vi "PC_Main.vi"() -> ()   [LabVIEW 2018]
uses:
  <vilib>/Analysis/Matrix/Datatypes/RealMatrix.ctl
  controls/Command.ctl
  <vilib>/Platform/TimedLoop/XDataNode/timing_clust.ctl
  <vilib>/Platform/TimedLoop/XDataNode/nitl_modes.ctl
  <vilib>/Platform/TimedLoop/XDataNode/wakeup.ctl
  <vilib>/Utility/error.llb/DialogType.ctl
  controls/Trial Config Settings.ctl
  controls/Command IN_Recipe.ctl
  controls/Rig Config Settings.ctl
  Globals/Global - Configuration Options.vi
  <vilib>/FPGAPlugInAG/cRIO-9045/niLvFpga_Open_cRIO-9045.vi
  <vilib>/rvi/interface/common/dynamic/niFpgaDynamicAddResources.vi
  <vilib>/Utility/error.llb/Error Cluster From Error Code.vi
  <vilib>/rvi/errors/niLvFpgaAdjustHostInterfaceError.vi
  <vilib>/measure/mascope.llb/Pulse Measurements 1 chan.vi
  <vilib>/FPGAPlugInAG/Dynamic/niLvFpga_Close_Dynamic.vi
  <vilib>/Platform/TimedLoop/XDataNode/XDataNode.xnode
  <vilib>/rvi/interface/nirviOpenFPGA/nirviOpenFPGA.xnode
  FPGA Bitfiles/UIUCWhiskerProje_FPGATarget_FPGABuild_ja8qmgOJlMY.lvbitx
  FPGA_Main.vi
  <vilib>/rvi/interface/nirviMethod/nirviMethod.xnode
  <vilib>/rvi/interface/nirviCloseFPGA/nirviCloseFPGA.xnode
  <vilib>/measure/NI_MAPro.lvlib
  <vilib>/Platform/TimedLoop/XDataNode/XDNodeRunTimeDep.lvlib
  <vilib>/FPGAPlugInAG/Dynamic/niLvFpga_ReadFifo_Dynamic.vi
  <vilib>/rvi/errors/niLvFpgaMergeErrorWithErrorCode.vi
  <vilib>/Analysis/Matrix/NI_Matrix.lvlib
panel:
  out "Start Test":bool=TRUE
  out "Plot Colors OUT":u32[](array[numeric])
  in  "Tab Control 2":enum32{"Misc", "Additional Graphs"}(tab)
  in  "Flash Drive Message":string="Reading Flash Drive...."
  in  "Water Delivery":bool
  in  "Water ON Time":i32=100
  out "# water":i32
  out "Watchdog Status":string
  out "# of CPUs":u32
  out "cRIO System Time":string
  out "cRIO System Date":string
  out "Real-Time Running?":bool caption="*Flashing LED means\nreal-time status is good"
  in  "Tree":string(tree)
  in  "Open Flash Drive Directory":bool
  in  "Refresh Tree":bool
  out "Test Folder":string
  in  "Slide":dbl(slide) min=-0.1 max=1.0 step=0.0025 scale=-0.1..1.0 scale format="%.3f"
  out "Histogram":dynamicdata(graph)
  out "XY Graph":cluster{dbl[], "Array 2":dbl[]}[](graph)
  in  "Histogram Plot2":u16(ring) items=["Habituation_20.dat"]
  in  "Histogram Plot1":u16(ring) items=["Habituation_20.dat"]
  out "Active Plots":i32
  in  "Enable Histogram?":bool=TRUE
  out "Lateral Trial History":dbl[][](array[numeric])
  in  "Save Data":bool=TRUE
  out "Drive Reconnect Message":string
  in  "Log Event":bool
  in  "View Event Log":bool
  in  "Error IN":errorcluster
  out "Error Out":errorcluster
  out "User Event":refnum<user-event>
  in  "Command":T1
  out "Status":string="Please Wait....."
  in  "Tab Control":T2(tab)
  in  "Group Size for Randomization":i32=1 min=1
  in  "Randomize Trials?":bool=TRUE
  in  "Load Default Sequence":bool
  in  "Save Trial Sequence":bool
  in  "Test Trials to Run":string[](array[combo])=["Left Turn.dat", "Right Turn.dat", "Straight.dat"]
  in  "Reset Sequence to Default":bool
  in  "History (Seconds):":dbl=20.0 format="%.1f"
  in  "X Axis (Seconds):":dbl=6.0 format="%.1f"
  out "Timeout Timer":dbl format="%.2f"
  out "cor_pos":sgl format="%.3f"
  out "cor_width":sgl
  out "Trial #":i32
  in  "Save Rig Sequence":bool
  in  "Test Rig Settings":string[](array[combo])=["Left Turn.dat", "Right Turn.dat", "Straight.dat"]
  in  "Rig editor":bool
  in  "Run #":string="02"
  in  "Animal #":string="0324810"
  in  "Date":string
  in  "Start Test":bool
  in  "Trial editor":bool
  out "Time Into Trial":dbl=4.01791524887085 format="%.2f"
  in  "Graph Update Interval":dbl=0.1 format="%.2f"
  out "Chart Ball Speed":cluster{dbl[], dbl[]}[](graph) caption="Ball Speed (Vball)"
  out "Test Trial In Progress":string
  out "Trial Tracker":string[][](table)=[["Test Reward.dat", "9", "8"], ["Test NO Reward.dat", "8", "0"]]
  out "Test In Progress":bool
  out "Trial Fraction":dbl format="%.6f"
  out "Total Test Time":dbl=4.01791524887085 format="%.2f"
  out "Graph X and Y Pos":cluster{"X":dbl, "Y":dbl}[](graph) caption="X and Y Position"
  out "Speed_Time_Length":i32
  out "mean_lat_vel":dbl
  out "mean_for_vel":dbl
  out "Vball":dbl format="%.3f"
  out "A_calib_matrix":T3
  out "for_ball_motion":dbl
  out "lat_ball_motion":dbl
  out "zero_V":T3
  out "cam_vel_ai_vlt":T3
  out "cam_vel_steps":T3
  out "step_V":dbl
  out "Frame Clock":waveform(i16)(graph)
  out "Freq":dbl caption="Hz"
  in  "Frame Clock Freq":dbl=500.0 caption="Hz"
  in  "laser_ON Time":i16=1 min=0
  in  "laser_OFF Time":i16=99 min=0
  in  "Digital Controls":bool[](array[boolean])=[FALSE, FALSE, FALSE, FALSE, FALSE, FALSE]
  in  "Send Digital Signals to FPGA":bool
  in  "Ephys Clock Freq":dbl=10000.0 caption="Hz"
  in  "Manual Override":bool
  in  "Analog Inputs_Override":sgl[](array[slide]) scale=-10.0..30.0
  out "LeftWall":dbl(slide)
  out "RightWall":dbl(slide) scale=0.0..25.0
  out "Cor_width_actual":dbl
  out "cor_width 2":sgl
  out "DIO":bool[](array[boolean])
  in  "Analog Outputs":sgl[](array[numeric])=[0.0, 0.0, 0.0, 0.0] min=0 max=5 format="%.5f"
  out "Analog Inputs":sgl[](array[numeric]) format="%.5f"
  in  "Exit":bool
  # "Behavioral Control Program v1.0.0.7"
  # "Default is 10Hz"
  # "Water Delivery"
  # "Real-Time OS"
  # "ms"
  # "File Name Variables"
  # "Trial Status"
  # "Mouse Speed"
  # "Trial Config"
  # "Mouse Lateral Position"
  # "Rig Config"
  # "Mouse Forward Position"
  # "*Change this setting via Rig Editor"
  # "secs"
  # "mm"
  # "mm"
  # "secs"
  # "secs"
  # "secs"
  # "*If Speed_Time_Length = 250\nthen averages are calculated every\n0.5 seconds since 1 data save takes\nplace every 0.002 seconds."
  # "="
  # "="
  # "avg"
  # "mean_for_vel"
  # "for_ball_motion (speed_time_length)"
  # "="
  # "="
  # "avg"
  # "mean_lat_vel"
  # "lat_ball_motion (speed_time_length)"
  # "cm/s"
  # "cm/s"
  # "2"
  # "2"
  # "="
  # "+"
  # "for_ball_motion"
  # "lat_ball_motion"
  # "cm/s"
  # "A_calib(0,0) x cam_vel_steps(0)"
  # "="
  # "A_calib(0,1) x cam_vel_steps(1)"
  # "cm/s"
  # "sum"
  # "A_calib(0,2) x cam_vel_steps(2)"
  # "A_calib(0,3) x cam_vel_steps(3)"
  # "A_calib(1,0) x cam_vel_steps(0)"
  # "="
  # "A_calib(1,1) x cam_vel_steps(1)"
  # "cm/s"
  # "sum"
  # "A_calib(1,2) x cam_vel_steps(2)"
  # "A_calib(1,3) x cam_vel_steps(3)"
  # "minus"
  # "="
  # "round"
  # "trial_ephys_ctrl"
  # "*this will trigger ephys_clock"
  # "whisker_video_ctrl"
  # "*this will trigger frame_clock"
  # "right_texture_ctrl"
  # "left_texture_ctrl"
  # "water_valve_ctrl"
  # "ON Time(msec)"
  # "OFF Time(msec)"
  # "laser_ctrl"
  # "*this will cycle the laser"
  # "laser"
  # "*this will cycle the laser voltage to the\namplitude called for using the analog\noutput labeled \"laser_AO3\" which is\nlocated on the Debug tab."
  # "Forward"
  # "Lateral"
  # "ANALOG OUTPUTS - Slot2"
  # "DIGITAL IO - Slot3"
  # "ANALOG INPUTS - Slot1"
  # "Chassis:  cRIO-9045"
  # "DIO0"
  # "aClck_DI"
  # "DIO1"
  # "frame_clock_DO"
  # "whisker_video_ctrl_DO"
  # "DIO2"
  # "DIO3"
  # "lick_signal_DO"
  # "water_valve_ctrl_DO"
  # "DIO4"
  # "DIO5"
  # "laser_ctrl"
  # "DIO6"
  # "left_texture_ctrl_DO"
  # "right_texture_ctrl_DO"
  # "DIO7"
  # "DIO8"
  # "trial_ephys_ctrl_DO"
  # "trial_iti_ctrl_DO"
  # "DIO9"
  # "trial_on_ctrl_DO"
  # "DIO10"
  # "ephys_clock_DO"
  # "DIO11"
  # "NI9403"
  # "left_wall_AO0"
  # "Vdc"
  # "right_wall_AO1"
  # "Vdc"
  # "AO2"
  # "Vdc"
  # "laser_AO3"
  # "Vdc"
  # "Vx0 raw Cam0"
  # "Vdc"
  # "Vdc"
  # "Vy0 raw Cam0"
  # "Vdc"
  # "Vx1 raw Cam1"
  # "Vy1 raw Cam1"
  # "Vdc"
  # "Software Installations"
  # "Flash Drive Setup"
  # "1) Labview 2018 w/f1 patch (32-bit)\n2) 2018 Labview Real-Time Module (32-bit)\n3) 2018 Labview FPGA Module (32-bit)\n4) DAQmx 18.0\n5) NI Compact RIO Drivers 18.1 (June 2018)\n6) 2018 XILINX 2017_2 (Compile Tools)"
  # "1) Make sure a fat32 formatted flash drive is inserted into the cRIO.\n\n2) Make sure the cRIO is mapped as a network drive on the main PC (see fig.1 below).  Webdav needs to be installed on the cRIO in order to do this. \n\n3) Make sure the correct path is entered in the Rig Config Settings for \"cRIO Test Data Dir\".  The flash drive will always be \"u\".  So, if the cRIO is mapped as network drive U then the correct path to put in the Rig Config Settings would be \"U:\\u\".\n\n4) Make sure the mapped network drive path is connected (figure 1).  If it isn't you will have to double click on the path at which point a login window will pop up.  Enter your Admin login and password.  If you do not have one then create one on the cRIO using via the \"Web Configuration\" page.  The default login for the cRIO is:   User name:  \"admin\"\n                                                                                                                 Password:  blank"
  # "*Install the above software packages in the order listed."
  # "Required Directories"
  # "C:\\Whisker Tester\\Rig\\\n*This directory will include 1) rig setup files (.dat) and 2) a default rig file (Sequence.xls) \n\nC:\\Whisker Tester\\Trials\\\n*This directory will include 1) trial setup files (.dat) and 2) a default trials list (Sequence.xls) \n\nC:\\Whisker Tester\\Event Logs\\\n*This directory will include event logs for various events that the developer wants to track (log.xls)"
  # "Figure 1 - cRIO Mapped Network Drive"
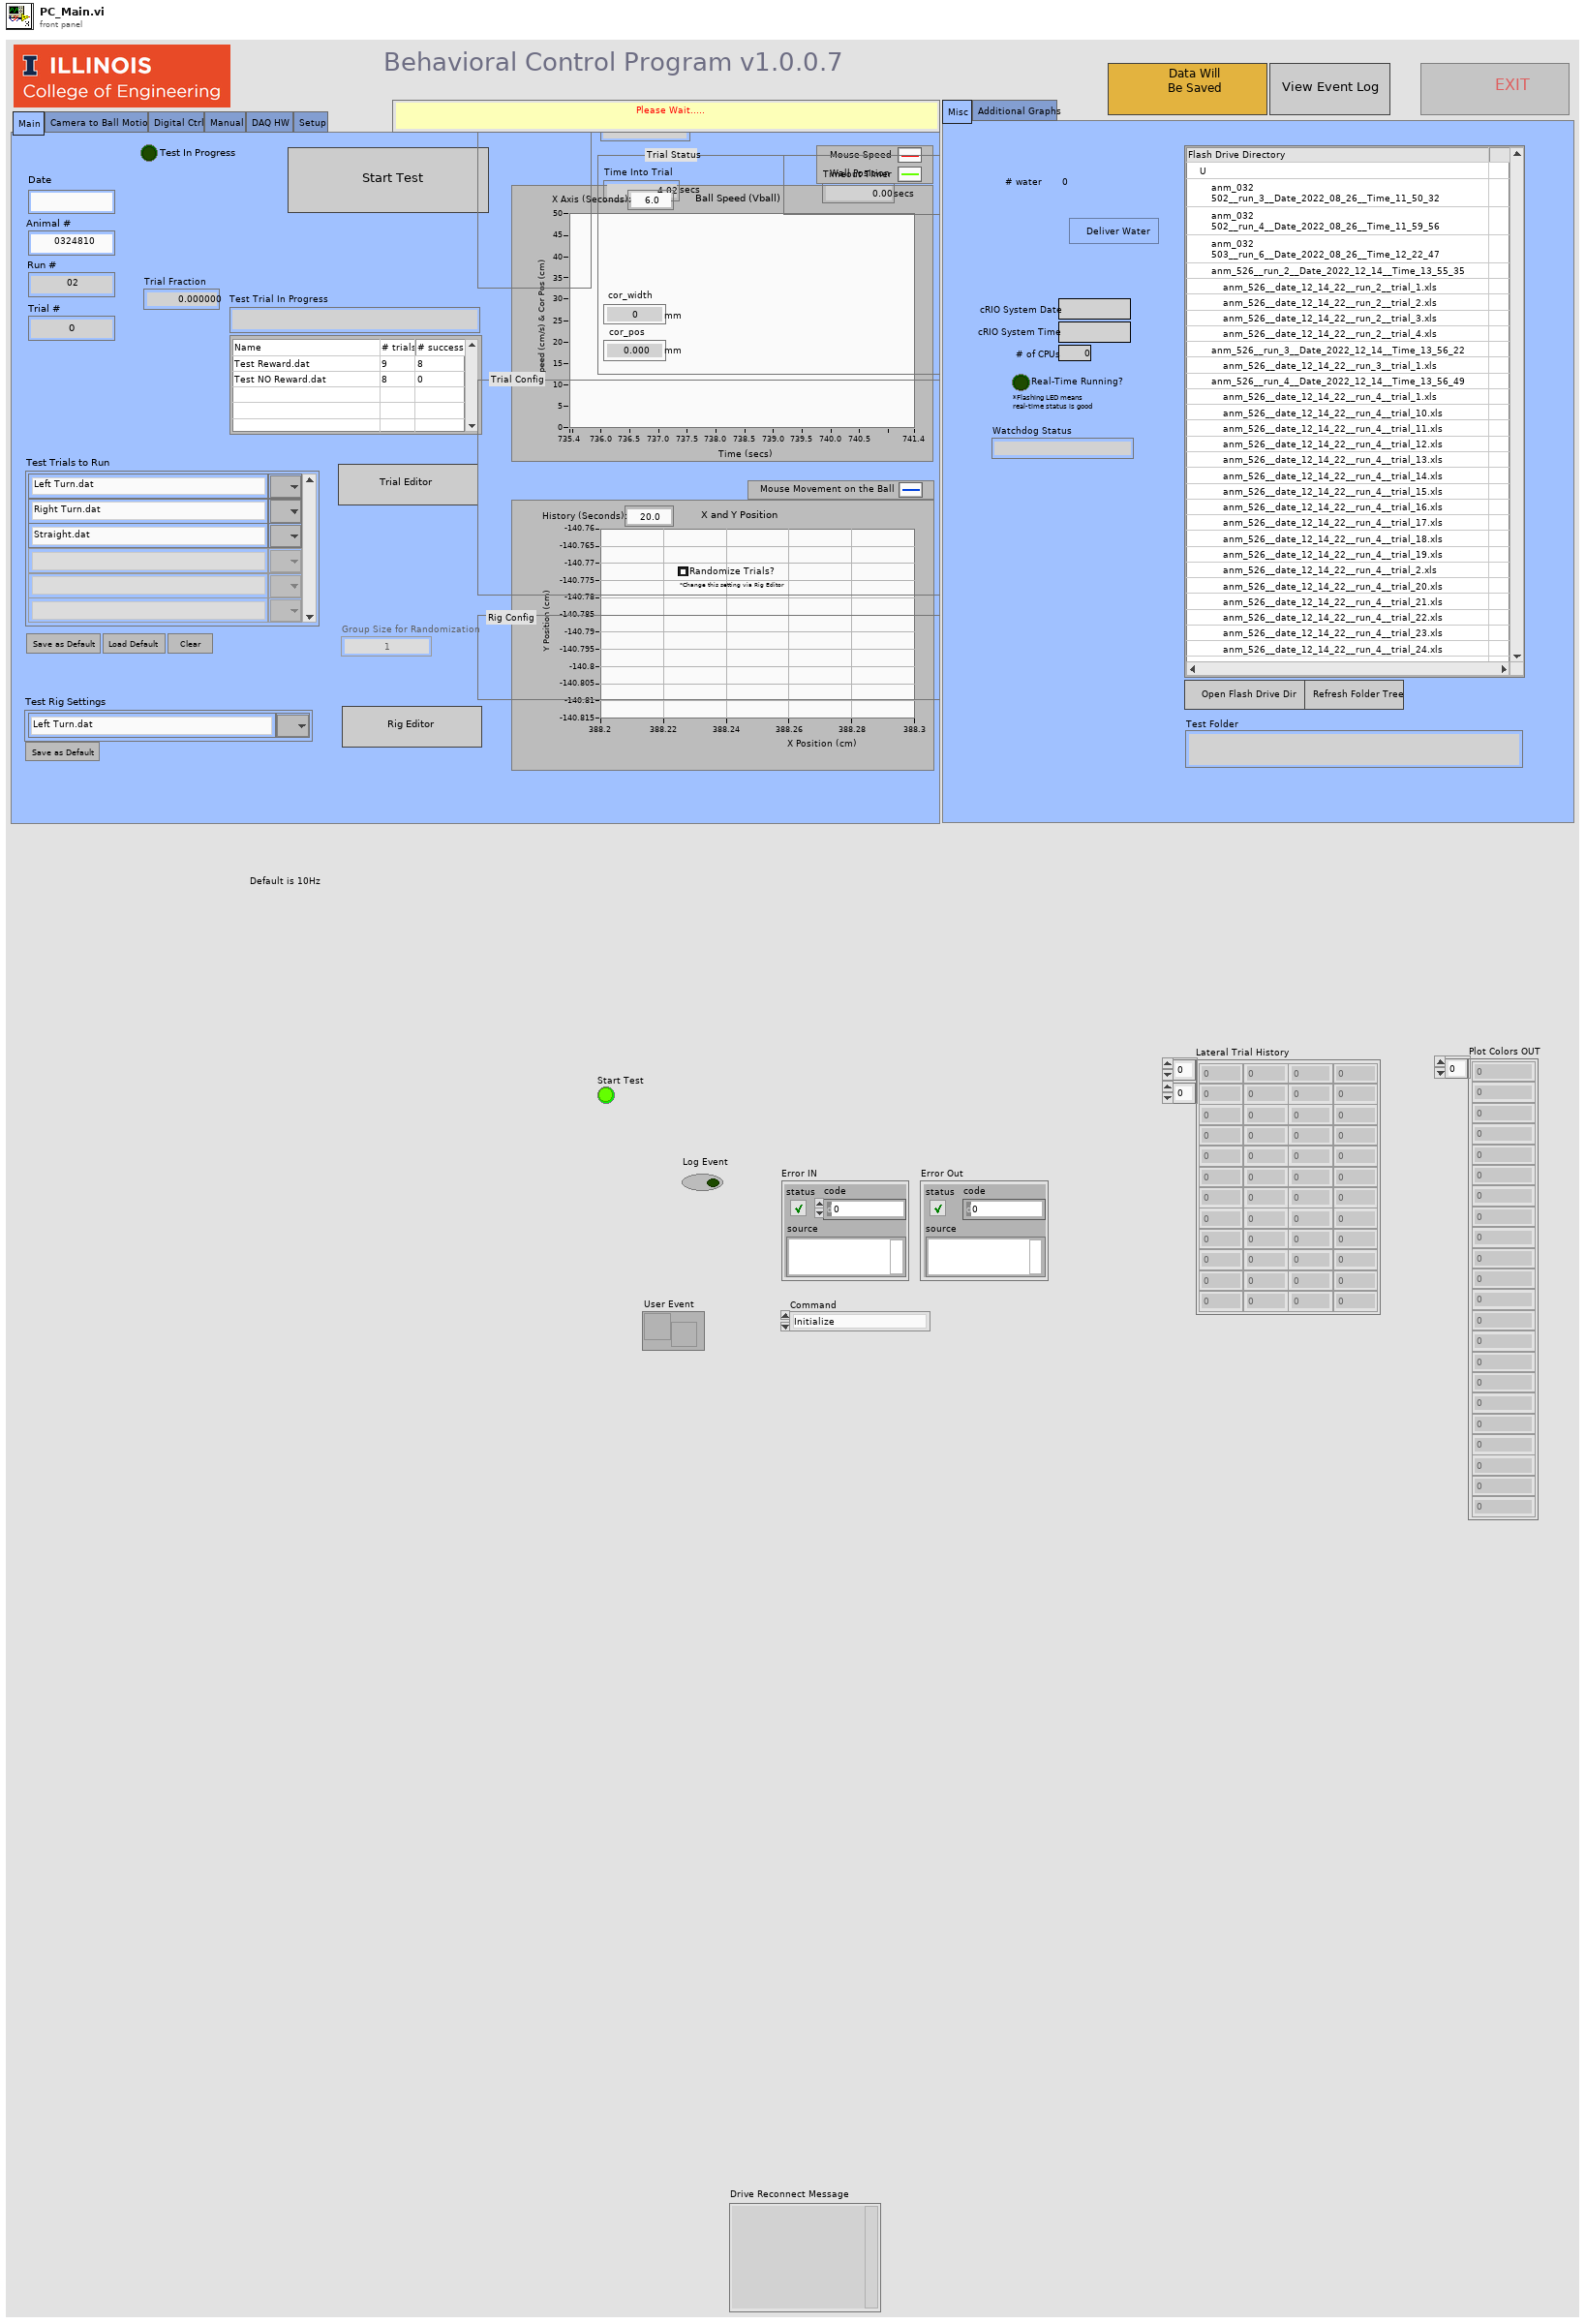
[diagram p1: front panel]
types:
  T1 = typedef "Command.ctl" = enum16{"Initialize", "Start Test", "Download All Trials to RT", "Water Delivery", "Rig Config Read", "cRIO Test Data Directory", "Update Folder Tree", "Log Event", "Abort", "Exit"}
  T2 = enum32{"Main", "Camera to Ball Motion", "Digital Ctrl", "Manual", "DAQ HW", "Setup"}
  T3 = typedef "NI_Matrix.lvlib/RealMatrix.ctl" = dbl[][]
  T4 = enum8{"Enabled", "Disabled", "Disabled and Grayed Out"}
  T5 = typedef "XDNodeRunTimeDep.lvlib/timing_clust.ctl" = cluster{"Expected End [f-1]":u64, "Actual End [f-1]":u64, "Finished Late? [f-1]":bool, "Expected End [i-1]":u64, "Actual End [i-1]":u64, "Finished Late? [i-1]":bool, "Expected Start [i]":u64, "Actual Start [i]":u64, "Expected Start [f]":u64, "Actual Start [f]":u64, "Source Name":string, "Structure Name":string, "Period":i64, "Deadline":i64, "Offset":i64, "Start":i64, "Priority":i32, "Timeout":i32, "Mode":T6, "Wakeup Reason":T7, "Error":errorcluster, "Source Type":string, "Secondary Source Type":string, "Global End Time":u64, "Global Start Time":u64, "Frame Duration":u64, "Iteration Duration":u64, "Assigned CPU":i32, "I/O Scan Engine Mode":u32}
  T6 = typedef "XDNodeRunTimeDep.lvlib/nitl_modes.ctl" = enum32{"No Change", "Process missed periods, maintain original phase", "Discard missed periods, maintain original phase", "Process missed periods, ignore original phase", "Discard missed periods, ignore original phase"}
  T7 = typedef "XDNodeRunTimeDep.lvlib/wakeup.ctl" = enum32{"Normal", "Aborted", "Asynchronous wakeup", "Timing source error", "Timed loop error", "Timeout"}
  T8 = typedef "Command IN_Recipe.ctl" = enum16{"Save", "Load"}
  T9 = enum32{"Page Enabled", "Page Disabled", "Page Disabled & Grayed"}
  T10 = enum32{"invalid app kind", "Development System", "Run Time System", "Student Edition", "Embedded LabVIEW", "Evaluation", "Custom"}
  T11 = typedef "DialogType.ctl" = u16
  T12 = typedef "Rig Config Settings.ctl" = cluster{"Rig Name":string, "Rig Room":string, "Base Directory":string, "Computer IP Address":string, "Globals Name":string, "Treatmill Str":string, "cRIO Test Data Dir":path, "ai":string, "ao":string, "dio":string, "A_calib_str_row1":string, "A_calib_str_row2":string, "A_calib_str_row3":string, "Zero_V_str":string, "step_V":string, "Sample Freq":string, "ai_threshold":string, "run_speed_thresh":string, "speed_time_length":string, "wall ball gain":string, "max wall pos":string, "max cor width":string, "Trial Config Directory":path, "Randomize Trials?":bool}
  T13 = typedef "Trial Config Settings.ctl" = cluster{"Trial Label":string, "Type":string, "Timeout (secs)":string, "Inter-Trial Interval (secs)":string, "Left Wall Enabled":bool, "Right Wall Enabled":bool, "Corridor Reset":bool, "Default Wall Position":string, "Open Loop Change Positions":string, "Open Loop Values (mm)":string, "Corridor Width Change Positions":string, "Corridor Width Values (mm) ":string, "Turn Change Positions":string, "Turn Values (deg)":string, "Left Texture Change Positions":string, "Right Texture Change Positions":string, "Video Frames (fps)":string, "Water Enabled":bool, "Water Trial Position":string, "Photostimulation":string, "Water Corridor Max":string, "Water Range":string, "Water Drop Size (ms)":string, "Water Reward Position":string, "Duration (cm)":string, "Left Texture Enabled":bool, "Right Texture Enabled":bool, "Ps Trial Period":string, "Ps Inter-Pulse-Interval (ms)":string, "Ps Peak Power":string, "Ps Pulse Duration (ms)":string, "ephys_clock freq (hz)":string, "frame_clock (hz)":string, "Plot Color (Lateral Dist vs Trial Fraction)":u32}
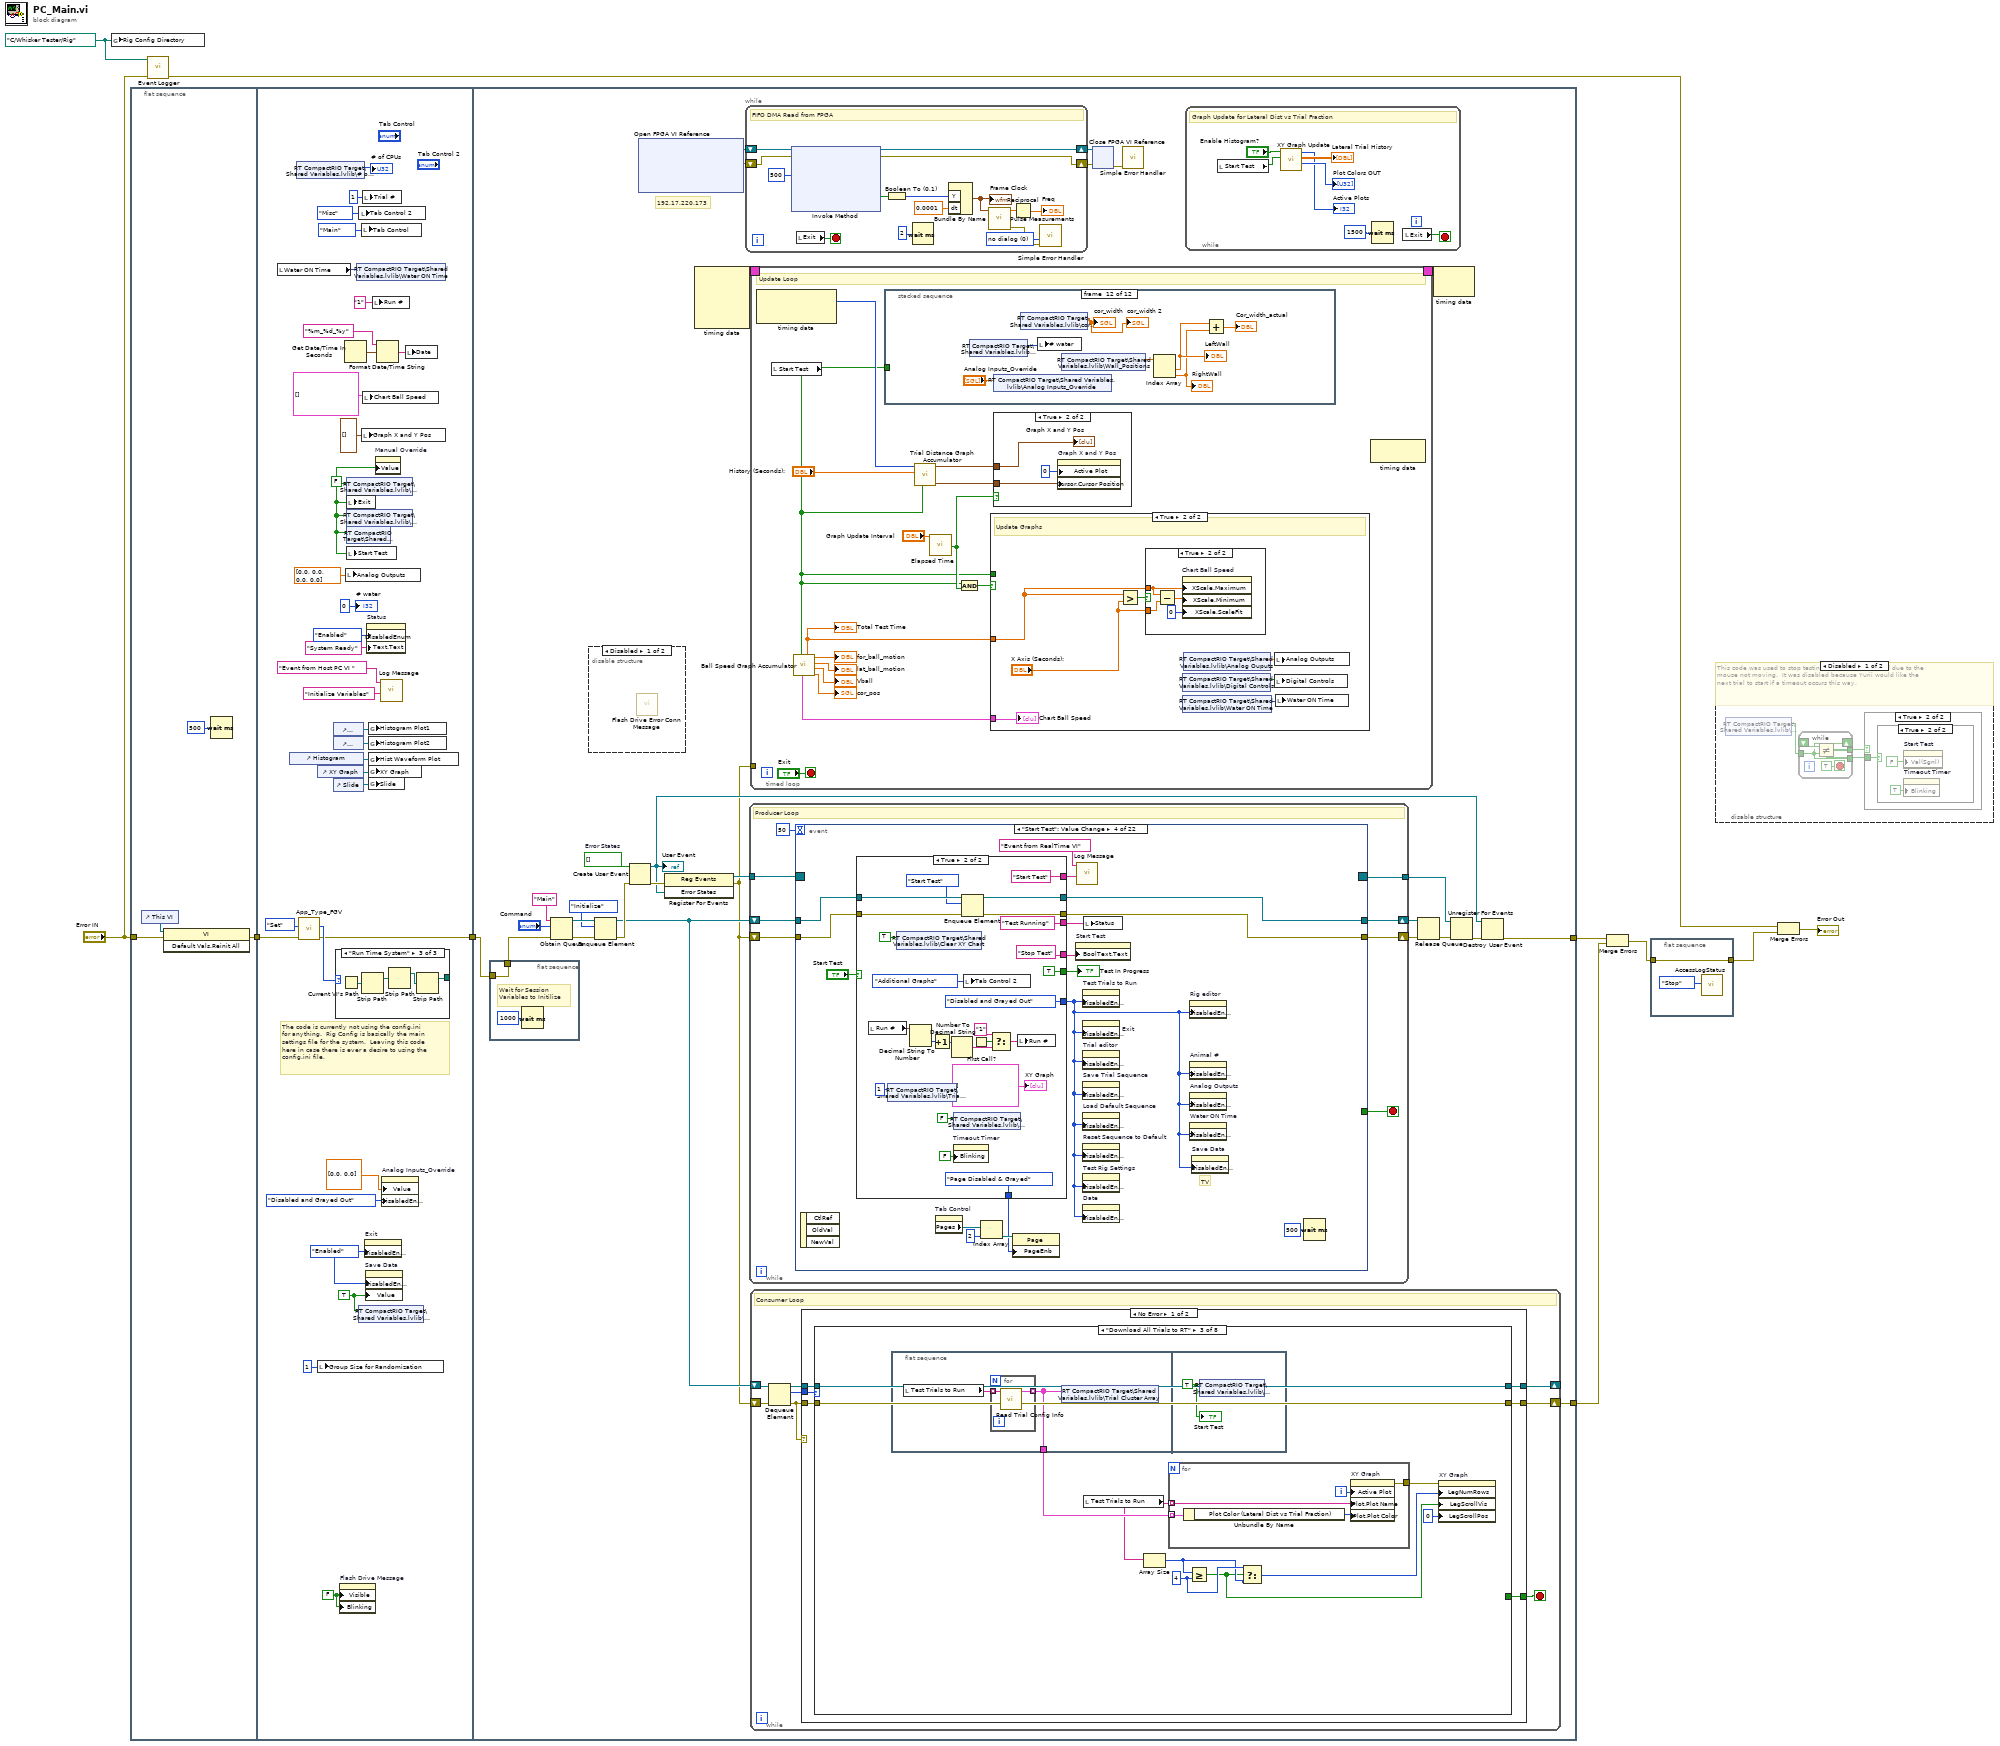
[diagram p0: block diagram]
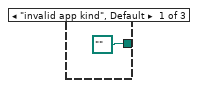
[diagram p5: hidden frame]
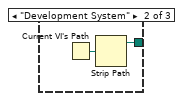
[diagram p6: hidden frame]
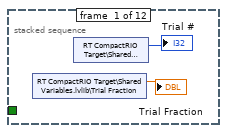
[diagram p8: hidden frame]
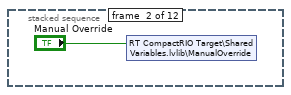
[diagram p9: hidden frame]
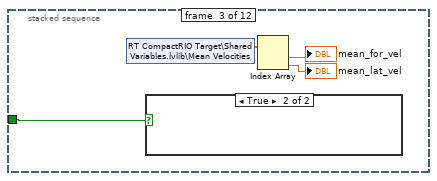
[diagram p10: hidden frame]
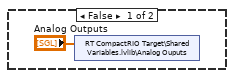
[diagram p11: hidden frame]
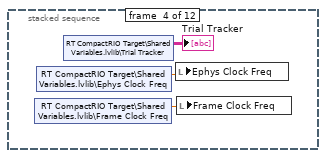
[diagram p12: hidden frame]
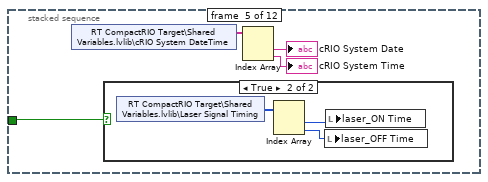
[diagram p13: hidden frame]
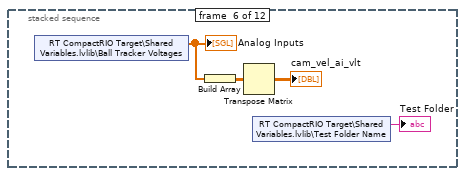
[diagram p15: hidden frame]
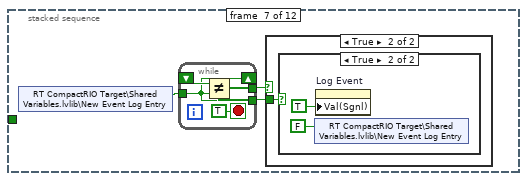
[diagram p16: hidden frame]
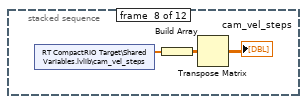
[diagram p19: hidden frame]
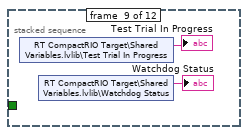
[diagram p20: hidden frame]
diagram:
  w5 = path "C:/Whisker Tester/Rig" ("Rig Config Directory")
  n1 = global write "Global - Configuration Options.vi" "Rig Config Directory"(w5) -> ()
  n2 = flat-sequence {
    tunnel: "Error IN" -> [w13]
    tunnel: [w12] -> w7
    tunnel: [w32] -> w8
    tunnel: w7 -> [w34]
    tunnel: [w66] -> w10
    tunnel: [w65] -> w9
    tunnel: w8 -> [w63]
    frame #0 {
      n3 = control-ref of="This VI"() -> (w14:refnum<vi>)
      n4 = invoke class="VI" method="Default Vals.Reinit All"(reference=w14, error in=w13) -> (error out=w12:errorcluster)  [unwired: 1 in, 2 out]
      n5 = Wait (ms)(milliseconds to wait=u32 500) -> ()  [unwired: 1 out]
    }
    frame #1 {
      w24 = FALSE ("Visible")
      w17 = T4."Enabled" ("Disabled")
      w16 = TRUE ("Save Data")
      w15 = FALSE ("New Trial Ready")
      # "The code is currently not using the config.ini\nfor anything.  Rig Config is basically the main\nsettings file for the system.  Leaving this code\nhere in case there is ever a desire to using the\nconfig.ini file."
      n6 = local read "Water ON Time"() -> (w44:i32)
      n7 = control-ref of="Histogram"() -> (w21:refnum<vi>)
      n8 = shared-variable "RT CompactRIO Target\\Shared Variables.lvlib\\# of CPUs"() -> (→"# of CPUs":u32)  [unwired: 1 in, 1 out]
      n9 = call "App_Type_FGV.vi"("error in"=w34, "Function"=enum16{"Get", "Set"}."Set") -> ("error out"=w32:errorcluster, "App. Type"=w33:T10)  [unwired: 8 in]
      n10 = control-ref of="XY Graph"() -> (w20:refnum<vi>)
      n11 = local write "Group Size for Randomization"(1 ("Group Size for Randomization")) -> ()
      n12 = control-ref of="Histogram Plot1"() -> (w22:refnum<vi>)
      n13 = control-ref of="Histogram Plot2"() -> (w23:refnum<vi>)
      n14 = control-ref of="Slide"() -> (w19:refnum<vi>)
      n15 = case shown="\"Run Time System\"" w33 {
        tunnel: [path "" ("stripped path") w49 w51] -> _
        frame "invalid app kind", Default {
        }
        frame "Development System" {
          n16 = Current VI's Path() -> (path=w50:path)
          n17 = Strip Path(path=w50) -> (stripped path=w49:path)  [unwired: 1 out]
        }
        frame "Run Time System" {
          n18 = Current VI's Path() -> (path=w52:path)
          n19 = Strip Path(path=w52) -> (stripped path=w53:path)  [unwired: 1 out]
          n20 = Strip Path(path=w53) -> (stripped path=w54:path)  [unwired: 1 out]
          n21 = Strip Path(path=w54) -> (stripped path=w51:path)  [unwired: 1 out]
        }
      }
      n22 = property on="Flash Drive Message" class="Str"("Visible"=w24, "Blinking"=w24) -> ()  [unwired: 2 in, 2 out]
      n23 = Get Date/Time In Seconds() -> (seconds since 1Jan1904=w47:timestamp)
      n24 = local write "Analog Outputs"(sgl[] [0.0, 0.0, 0.0, 0.0] ("Analog Outputs")) -> ()
      n25 = shared-variable "RT CompactRIO Target\\Shared Variables.lvlib\\Start Test"(w15) -> ()  [unwired: 1 in, 1 out]
      n26 = local write "Exit"(w15) -> ()
      n27 = shared-variable "RT CompactRIO Target\\Shared Variables.lvlib\\Timeout?"(w15) -> ()  [unwired: 1 in, 1 out]
      n28 = shared-variable "RT CompactRIO Target\\Shared Variables.lvlib\\Exit"(w15) -> ()  [unwired: 1 in, 1 out]
      n29 = local write "Start Test"(w15) -> ()
      n30 = shared-variable "RT CompactRIO Target\\Shared Variables.lvlib\\Water ON Time"(w44) -> ()  [unwired: 1 in, 1 out]
      n31 = local write "Tab Control 2"(enum32{"Misc", "Additional Graphs"}."Misc" ("Tab Control 2")) -> ()
      n32 = shared-variable "RT CompactRIO Target\\Shared Variables.lvlib\\SaveData"(w16) -> ()  [unwired: 1 in, 1 out]
      n33 = local write "Tab Control"(T2."Main" ("Tab Control")) -> ()
      n34 = local write "Graph X and Y Pos"(cluster{"X":dbl, "Y":dbl}[] [] ("XY Graph")) -> ()
      n35 = local write "Trial #"(1 ("Trial #")) -> ()
      n36 = local write "Chart Ball Speed"(cluster{dbl[], dbl[]}[] [] ("Chart Ball Speed")) -> ()
      n37 = property on="Exit" class="Bool (strict)"("DisabledEnum"=w17) -> ()  [unwired: 2 in, 2 out]
      n38 = property on="Save Data" class="Bool (strict)"("DisabledEnum"=w17, "Value"=w16) -> ()  [unwired: 2 in, 2 out]
      n39 = property on="Status" class="Str"("DisabledEnum"=T4."Enabled" ("Disabled"), "Text.Text"="System Ready" ("Status")) -> ()  [unwired: 2 in, 2 out]
      n40 = global write "Global - Configuration Options.vi" "Histogram Plot1"(w22) -> ()
      n41 = global write "Global - Configuration Options.vi" "Histogram Plot2"(w23) -> ()
      n42 = global write "Global - Configuration Options.vi" "Hist Waveform Plot"(w21) -> ()
      n43 = global write "Global - Configuration Options.vi" "XY Graph"(w20) -> ()
      n44 = global write "Global - Configuration Options.vi" "Slide"(w19) -> ()
      n45 = local write "Run #"("1" ("Run #")) -> ()
      n46 = property on="Manual Override" class="Bool (strict)"("Value"=w15) -> ()  [unwired: 2 in, 2 out]
      n47 = Format Date/Time String(time format string (%c)="%m_%d_%y", seconds (now)=w47) -> (date/time string=w45:string)  [unwired: 1 in]
      n48 = call "Log Message.vi"("Message"="Initialize Variables", "Log Type"="Event from Host PC VI ") -> ()  [unwired: 8 in, 2 out]
      n49 = property on="Analog Inputs_Override" class="Arr (strict)"("Value"=sgl[] [0.0, 0.0] ("Analog Inputs_Override"), "DisabledEnum"=T4."Disabled and Grayed Out" ("Disabled")) -> ()  [unwired: 2 in, 2 out]
      n50 = local write "Date"(w45) -> ()
      "# water" <- 0 ("# water")
    }
    frame #2 {
      w70 = bool[] []  # Error States
      # "192.17.220.173"
      n51 = flat-sequence {
        tunnel: w63 -> [w192]
        tunnel: [w192] -> w62
        frame #0 {
          # "Wait for Session\nVariables to Initilize"
          n52 = Wait (ms)(milliseconds to wait=u32 1000) -> ()  [unwired: 1 out]
        }
      }
      n53 = Obtain Queue(name (unnamed)="Main", element data type="Command", error in (no error)=w62) -> (queue out=w79:refnum<queue>, error out=w78:errorcluster)  [unwired: 2 in, 1 out]
      n54 = disable-structure shown="Disabled" {
        frame Disabled {
          n55 = call "Flash Drive Error Conn Message.vi"() -> ()  [unwired: 12 in]
        }
        frame Enabled {
        }
      }
      n56 = Enqueue Element(queue=w79, element=Command."Initialize", error in (no error)=w78) -> (queue out=w68:refnum<queue>, error out=w80:errorcluster)  [unwired: 1 in, 1 out]
      n57 = Create User Event(user event datatype=w70, error in=w80) -> (user event=w71:refnum<user-event>, error out=w81:errorcluster)
      "User Event" <- w71
      n58 = xnode "Open FPGA VI Reference"() -> ("FPGA VI Reference Out"=w59:refnum<k20>, "error out"=w55:errorcluster)  [unwired: 2 in]
      n59 = register-events(error in=w81, w71) -> (reference out=w82:refnum<event-registration>, error out=w64:errorcluster)  [unwired: 1 in]
      n60 = node-c288() -> (w61:T5)  [unwired: 4 in]
      n61 = while {
        shift-right: [w94] -> w57
        shift-left: w59 -> [w97]
        shift-right: [w93] -> w56
        shift-left: w55 -> [w92]
        stop <- w96 stop-if-true
        w84 = T11 0 items=["no dialog", "OK message", "continue or stop message", "OK message + warnings", "continue/stop + warnings"] ("type of dialog (OK msg:1)")
        # "FIFO DMA Read from FPGA"
        n62 = xnode "Invoke Method"("FPGA VI Reference In"=w97, "error in"=w92, "Number of Elements"=u32 500) -> ("FPGA VI Reference Out"=w94:refnum<k20>, "error out"=w93:errorcluster, "Data"=w89:bool[])  [unwired: 1 in, 1 out]
        n63 = local read "Exit"() -> (w96:bool)
        n64 = Boolean To (0,1)(Boolean=w89) -> (0, 1=w90:i16[])
        n65 = Wait (ms)(milliseconds to wait=u32 2) -> ()  [unwired: 1 out]
        n66 = Bundle By Name("Y"=w90, "dt"=0.0001) -> (w87:waveform(i16))  [unwired: 1 in]
        "Frame Clock" <- w87
        n67 = call-poly <vilib>:"Pulse Measurements.vi"("signal in"=w87) -> ("error out"=w85:errorcluster, "period"=w88:dbl)  [unwired: 6 in, 3 out]
        n68 = Reciprocal(x=w88) -> (1/x=→"Freq":dbl)
        n69 = call <vilib>:"Simple Error Handler.vi"("type of dialog (OK msg:1)"=w84, "error in (no error)"=w85) -> ()  [unwired: 3 in, 5 out]
      }
      n70 = while {
        tunnel: w82 -> [w429]
        shift-right: [w425] -> w74
        shift-left: w68 -> [w427]
        shift-right: [w424] -> w73
        shift-left: w64 -> [w426]
        tunnel: [w428] -> w72
        stop <- w430 stop-if-true
        # "Producer Loop"
        n71 = event shown="[3] \"Start Test\": Value Change" {
          selector: w429 -> [_ _ _ _ _ _ _ _ _ _ _ _ _ _ _ _ _ _ _ _ _ _]
          dyn-events: [_ _ _ _ _ _ _ _ _ _ _ _ _ _ _ _ _ _ _ _ _ _] -> w428
          timeout: 50 -> [_ _ _ _ _ _ _ _ _ _ _ _ _ _ _ _ _ _ _ _ _ _]
          tunnel: [_ _ _ _ _ _ _ _ _ _ _ _ _ _ _ _ _ _ _ _ _ TRUE] -> w430
          tunnel: w427 -> [w432 w434 w441 w458 w504 w509 w516 w522 w527 w537 w539 w542 w548 w553 w569 w572 w601 w614 w622 w625 w630 w635]
          tunnel: w426 -> [w431 w433 w440 w456 w503 w508 w515 w521 w526 w536 w538 w541 w547 w552 w566 w571 w600 w613 w621 w624 w629 w634]
          tunnel: [w432 w434 w441 w457 w504 w509 w516 w520 w527 w537 w539 w542 w548 w551 w568 w572 w601 w614 w620 w625 w630 w633] -> w425
          tunnel: [w431 w433 w440 w455 w503 w508 w514 w519 w526 w536 w538 w541 w547 w550 w567 w571 w600 w613 w619 w624 w629 w632] -> w424
          event Timeout {
            n72 = event-data() -> ()  [unwired: 1 in, 3 out]
          }
          event "Save Trial Sequence": Value Change {
            n73 = event-data() -> ()  [unwired: 1 in, 6 out]
            n74 = flat-sequence {
              frame #0 {
                n75 = call "Sequence Read_Write.vi"("Trial or Rig"=enum16{"Trial", "Rig"}."Trial", "Sequence IN"="Test Trials to Run", "Select"=enum16{"Save Sequence", "Read Sequence"}."Save Sequence") -> ()  [unwired: 7 in, 2 out]
              }
              frame #1 {
                n76 = Wait (ms)(milliseconds to wait=u32 500) -> ()  [unwired: 1 out]
              }
              frame #2 {
                n77 = local write "Save Trial Sequence"(FALSE ("Save Sequence")) -> ()
              }
            }
          }
          event "Save Rig Sequence": Value Change {
            n78 = event-data() -> ()  [unwired: 1 in, 6 out]
            n79 = flat-sequence {
              frame #0 {
                n80 = call "Sequence Read_Write.vi"("Trial or Rig"=enum16{"Trial", "Rig"}."Rig", "Sequence IN"="Test Rig Settings", "Select"=enum16{"Save Sequence", "Read Sequence"}."Save Sequence") -> ()  [unwired: 7 in, 2 out]
              }
              frame #1 {
                n81 = Wait (ms)(milliseconds to wait=u32 500) -> ()  [unwired: 1 out]
              }
              frame #2 {
                n82 = local write "Save Rig Sequence"(FALSE ("Save Sequence")) -> ()
              }
            }
          }
          event "Start Test": Value Change {
            # "TV"
            n83 = event-data() -> ()  [unwired: 1 in, 3 out]
            n84 = case shown="True" "Start Test" {
              tunnel: [T4."Enabled" ("Disabled") T4."Disabled and Grayed Out" ("Disabled")] -> w447
              tunnel: ["Start Test" ("Boolean Text.Text") "Stop Test" ("Boolean Text.Text")] -> w461
              tunnel: [FALSE ("Start Test") TRUE ("Start Test")] -> w460
              tunnel: ["Test Stopped" ("Status") "Test Running" ("Status")] -> w459
              tunnel: w458 -> [w467 w497]
              tunnel: [w465 w496] -> w457
              tunnel: w456 -> [w466 w494]
              tunnel: [w464 w493] -> w455
              tunnel: [T9."Page Enabled" ("Page Enabled State") T9."Page Disabled & Grayed" ("Page Enabled State")] -> w451
              tunnel: ["Stop Test" ("Message") "Start Test" ("Message")] -> w450
              frame False {
                n85 = stacked-sequence {
                  frame #0 {
                    w474 = FALSE ("Start Test")
                    n86 = shared-variable "RT CompactRIO Target\\Shared Variables.lvlib\\Start Test"(w474) -> ()  [unwired: 1 in, 1 out]
                    n87 = local write "Start Test"(w474) -> ()
                  }
                  frame #1 {
                    # "Give Real-Time VI time to\nhandle this manual test stop\nfrom this Host VI."
                    n88 = Wait (ms)(milliseconds to wait=u32 100) -> ()  [unwired: 1 out]
                  }
                  frame #2 {
                    w476 = bool[] [FALSE, FALSE, FALSE, FALSE, FALSE, FALSE] ("Digital Controls")
                    n89 = local write "Analog Outputs"(sgl[] [0.0, 0.0, 0.0, 0.0] ("Analog Outputs")) -> ()
                    n90 = local write "Digital Controls"(w476) -> ()
                    n91 = shared-variable "RT CompactRIO Target\\Shared Variables.lvlib\\Digital Controls"(w476) -> ()  [unwired: 1 in, 1 out]
                  }
                }
                n92 = Enqueue Element(queue=w467, element=Command."Update Folder Tree", error in (no error)=w466) -> (queue out=w465:refnum<queue>, error out=w464:errorcluster)  [unwired: 1 in, 1 out]
              }
              frame True {
                n93 = local read "Run #"() -> (w484:string)
                n94 = shared-variable "RT CompactRIO Target\\Shared Variables.lvlib\\Trial Index"(1 ("Trial Index")) -> ()  [unwired: 1 in, 1 out]
                n95 = shared-variable "RT CompactRIO Target\\Shared Variables.lvlib\\Clear XY Chart"(TRUE ("Clear XY Chart")) -> ()  [unwired: 1 in, 1 out]
                n96 = Decimal String To Number(string=w484) -> (number=w483:i32)  [unwired: 2 in, 1 out]
                n97 = Increment(x=w483) -> (x+1=w482:i32)
                n98 = Number To Decimal String(number=w482) -> (decimal integer string=w481:string)  [unwired: 1 in]
                n99 = property on="Timeout Timer" class="DigNum (strict)"("Blinking"=FALSE) -> ()  [unwired: 2 in, 2 out]
                n100 = shared-variable "RT CompactRIO Target\\Shared Variables.lvlib\\Timeout?"(FALSE ("Timeout?")) -> ()  [unwired: 1 in, 1 out]
                n101 = Enqueue Element(queue=w497, element=Command."Start Test", error in (no error)=w494) -> (queue out=w496:refnum<queue>, error out=w493:errorcluster)  [unwired: 1 in, 1 out]
                n102 = local write "Tab Control 2"(enum32{"Misc", "Additional Graphs"}."Additional Graphs" ("Tab Control 2")) -> ()
                n103 = First Call?() -> (First Call?: T/F=w487:bool)
                n104 = Select(t="1" ("Boolean Text.Text"), s=w487, f=w481) -> (s? t:f=w485:string)
                n105 = local write "Run #"(w485) -> ()
                "XY Graph" <- cluster{dbl[], "Array 2":dbl[]}[] [] ("XY Graph")
              }
            }
            "Test In Progress" <- w460
            n106 = property on="Tab Control" class="TabCtl (strict)"() -> ("Pages"=w453:refnum<vi>[])  [unwired: 2 in, 2 out]
            n107 = Index Array(array=w453, index=2) -> (element=w454:refnum<vi>)
            n108 = property class="Page"(reference=w454, "PageEnb"=w451) -> ()  [unwired: 1 in, 2 out]
            n109 = property on="Start Test" class="Bool (strict)"("BoolText.Text"=w461) -> ()  [unwired: 2 in, 2 out]
            n110 = call "Log Message.vi"("Message"=w450, "Log Type"="Event from RealTime VI") -> ()  [unwired: 8 in, 2 out]
            n111 = property on="Test Trials to Run" class="Arr (strict)"("DisabledEnum"=w447) -> ()  [unwired: 2 in, 2 out]
            n112 = property on="Exit" class="Bool (strict)"("DisabledEnum"=w447) -> ()  [unwired: 2 in, 2 out]
            n113 = property on="Trial editor" class="Bool (strict)"("DisabledEnum"=w447) -> ()  [unwired: 2 in, 2 out]
            n114 = property on="Save Trial Sequence" class="Bool (strict)"("DisabledEnum"=w447) -> ()  [unwired: 2 in, 2 out]
            n115 = property on="Load Default Sequence" class="Bool (strict)"("DisabledEnum"=w447) -> ()  [unwired: 2 in, 2 out]
            n116 = property on="Reset Sequence to Default" class="Bool (strict)"("DisabledEnum"=w447) -> ()  [unwired: 2 in, 2 out]
            n117 = property on="Test Rig Settings" class="Arr (strict)"("DisabledEnum"=w447) -> ()  [unwired: 2 in, 2 out]
            n118 = property on="Date" class="Str"("DisabledEnum"=w447) -> ()  [unwired: 2 in, 2 out]
            n119 = local write "Status"(w459) -> ()
            n120 = property on="Rig editor" class="Bool (strict)"("DisabledEnum"=w447) -> ()  [unwired: 2 in, 2 out]
            n121 = property on="Animal #" class="Str"("DisabledEnum"=w447) -> ()  [unwired: 2 in, 2 out]
            n122 = property on="Analog Outputs" class="Arr (strict)"("DisabledEnum"=w447) -> ()  [unwired: 2 in, 2 out]
            n123 = property on="Water ON Time" class="DigNum (strict)"("DisabledEnum"=w447) -> ()  [unwired: 2 in, 2 out]
            n124 = property on="Save Data" class="Bool (strict)"("DisabledEnum"=w447) -> ()  [unwired: 2 in, 2 out]
            n125 = Wait (ms)(milliseconds to wait=u32 500) -> ()  [unwired: 1 out]
          }
          event "Slide": Mouse Up {
            n126 = event-data() -> ()  [unwired: 1 in, 4 out]
            n127 = local read "Enable Histogram?"() -> (w502:bool)
            n128 = case shown="True" w502 {
              frame False {
              }
              frame True {
                n129 = shared-variable "RT CompactRIO Target\\Shared Variables.lvlib\\Test Trial Plot Color Array"() -> (w507:u32[])  [unwired: 1 in, 1 out]
                n130 = shared-variable "RT CompactRIO Target\\Shared Variables.lvlib\\Lateral Trial History"() -> (w506:dbl[][])  [unwired: 1 in, 1 out]
                n131 = call "Histogram Update.vi"("Lat Hist at Trial Fraction"=w506, "Test Trial Plot Color Array IN"=w507, "Trial Fraction Interval"=0.0025 ("y")) -> ()  [unwired: 12 in, 5 out]
              }
            }
          }
          event "Slide": Value Change {
            n132 = event-data() -> ()  [unwired: 1 in, 6 out]
            n133 = property on="XY Graph" class="XYGraph (strict)"("Active Cursor"=u32 0, "Cursor.Cursor X"="Slide", "Cursor.Cursor Y"=-10.0 ("Cursor.Cursor Position:Cursor Y")) -> ()  [unwired: 2 in, 2 out]
          }
          event "View Event Log": Value Change {
            n134 = event-data() -> ()  [unwired: 1 in, 6 out]
            n135 = call "Popup - Event Log Viewer.vi"("Error IN"=w515) -> ("Error OUT"=w513:errorcluster)  [unwired: 10 in]
            n136 = flat-sequence {
              tunnel: w513 -> [w517]
              tunnel: [w517] -> w514
              frame #0 {
                n137 = local write "View Event Log"(FALSE ("View Event Log")) -> ()
              }
            }
          }
          event "Open Flash Drive Directory": Value Change {
            n138 = event-data() -> ()  [unwired: 1 in, 6 out]
            n139 = Enqueue Element(queue=w522, element=Command."cRIO Test Data Directory", error in (no error)=w521) -> (queue out=w520:refnum<queue>, error out=w519:errorcluster)  [unwired: 1 in, 1 out]
          }
          event "Send Digital Signals to FPGA": Value Change {
            n140 = event-data() -> ()  [unwired: 1 in, 6 out]
            n141 = stacked-sequence {
              frame #0 {
                n142 = Build Array("laser_ON Time", "laser_OFF Time") -> (w532:i16[])
                n143 = shared-variable "RT CompactRIO Target\\Shared Variables.lvlib\\Ephys Clock Freq"("Ephys Clock Freq") -> ()  [unwired: 1 in, 1 out]
                n144 = shared-variable "RT CompactRIO Target\\Shared Variables.lvlib\\Frame Clock Freq"("Frame Clock Freq") -> ()  [unwired: 1 in, 1 out]
                n145 = shared-variable "RT CompactRIO Target\\Shared Variables.lvlib\\Laser Signal Timing"(w532) -> ()  [unwired: 1 in, 1 out]
              }
              frame #1 {
                n146 = Wait (ms)(milliseconds to wait=u32 500) -> ()  [unwired: 1 out]
              }
              frame #2 {
                n147 = local write "Send Digital Signals to FPGA"(FALSE ("Send Digital Signals to FPGA")) -> ()
              }
            }
            n148 = shared-variable "RT CompactRIO Target\\Shared Variables.lvlib\\Digital Controls"("Digital Controls") -> ()  [unwired: 1 in, 1 out]
            n149 = property on="Send Digital Signals to FPGA" class="Bool (strict)"("DisabledEnum"=T4."Disabled and Grayed Out" ("Disabled")) -> ()  [unwired: 2 in, 2 out]
          }
          event "Digital Controls", "Ephys Clock Freq", "Frame Clock Freq", "laser_OFF Time", "laser_ON Time": Value Change {
            n150 = event-data() -> ()  [unwired: 1 in, 6 out]
            n151 = property on="Send Digital Signals to FPGA" class="Bool (strict)"("DisabledEnum"=T4."Enabled" ("Disabled")) -> ()  [unwired: 2 in, 2 out]
          }
          event "Trial editor": Value Change {
            n152 = event-data() -> ()  [unwired: 1 in, 6 out]
            n153 = flat-sequence {
              frame #0 {
                n154 = call "Trial - Editor.vi"() -> ()  [unwired: 11 in, 1 out]
              }
              frame #1 {
                n155 = local write "Trial editor"(FALSE ("Trial editor")) -> ()
              }
            }
          }
          event "Manual Override": Value Change {
            n156 = event-data() -> ("NewVal"=w543:bool)  [unwired: 1 in, 5 out]
            n157 = case shown="False" w543 {
              frame False {
                n158 = property on="Analog Inputs_Override" class="Arr (strict)"("Value"=sgl[] [0.0, 0.0] ("Analog Inputs_Override"), "DisabledEnum"=T4."Disabled and Grayed Out" ("Disabled")) -> ()  [unwired: 2 in, 2 out]
              }
              frame True {
                n159 = property on="Analog Inputs_Override" class="Arr (strict)"("DisabledEnum"=T4."Enabled" ("Disabled")) -> ()  [unwired: 2 in, 2 out]
              }
            }
          }
          event "Save Data": Value Change {
            n160 = event-data() -> ("NewVal"=w549:bool)  [unwired: 1 in, 5 out]
            n161 = shared-variable "RT CompactRIO Target\\Shared Variables.lvlib\\SaveData"(w549) -> ()  [unwired: 1 in, 1 out]
          }
          event "Rig editor": Value Change {
            n162 = event-data() -> ()  [unwired: 1 in, 6 out]
            n163 = stacked-sequence {
              tunnel: w553 -> [_ _ w563 _]
              tunnel: w552 -> [_ _ w562 _]
              tunnel: [_ _ w561 _] -> w551
              tunnel: [_ _ w560 _] -> w550
              frame #0 {
                n164 = call "Rig - Editor.vi"() -> ()  [unwired: 11 in, 1 out]
              }
              frame #1 {
                n165 = global read "Global - Configuration Options.vi" "Rig Config Settings"() -> (w559:T12)
                n166 = Unbundle By Name(w559) -> ("Randomize Trials?"=w554:bool)
                n167 = local write "Randomize Trials?"(w554) -> ()
                n168 = Select(t=T4."Enabled" ("Disabled"), s=w554, f=T4."Disabled and Grayed Out" ("Disabled")) -> (s? t:f=w558:T4)
                n169 = property on="Group Size for Randomization" class="DigNum (strict)"("DisabledEnum"=w558, "Value"=1 ("Group Size for Randomization")) -> ()  [unwired: 2 in, 2 out]
              }
              frame #2 {
                n170 = Enqueue Element(queue=w563, element=Command."Rig Config Read", error in (no error)=w562) -> (queue out=w561:refnum<queue>, error out=w560:errorcluster)  [unwired: 1 in, 1 out]
              }
              frame #3 {
                n171 = local write "Rig editor"(FALSE ("Trial editor")) -> ()
              }
            }
          }
          event "Refresh Tree": Value Change {
            n172 = event-data() -> ()  [unwired: 1 in, 6 out]
            n173 = Enqueue Element(queue=w569, element=Command."Update Folder Tree", error in (no error)=w566) -> (queue out=w568:refnum<queue>, error out=w567:errorcluster)  [unwired: 1 in, 1 out]
          }
          event "Load Default Sequence": Value Change {
            n174 = event-data() -> ()  [unwired: 1 in, 6 out]
            n175 = stacked-sequence {
              seq-local: [w573 _ _ _] -> [_ _ _ w586]
              frame #0 {
                w578 = refnum<vi> refnum  # ComboBox
                n176 = control-ref of="Test Trials to Run"() -> (w579:refnum<vi>)
                n177 = invoke class="Arr (strict)" method="Reinit To Default"(reference=w579) -> (error out=w575:errorcluster)  [unwired: 2 in, 2 out]
                n178 = property on="Test Trials to Run" class="Arr (strict)"(error in=w575) -> (error out=w574:errorcluster, "Array Element"=w577:refnum<vi>)  [unwired: 1 in, 1 out]
                n179 = call "Trial Config - Load Filenames.vi"() -> ("Trial Config File Names OUT"=w573:string[])  [unwired: 10 in, 1 out]
                n180 = To More Specific Class(target class=w578, reference=w577) -> (specific class reference=w576:refnum<vi>)  [unwired: 1 in, 1 out]
                n181 = property class="CmbBox"(reference=w576, error in=w574, "Strings[]"=w573) -> ()  [unwired: 2 out]
              }
              frame #1 {
                n182 = Wait (ms)(milliseconds to wait=u32 500) -> ()  [unwired: 1 out]
              }
              frame #2 {
                n183 = local write "Load Default Sequence"(FALSE ("Load Default Sequence")) -> ()
              }
              frame #3 {
                # "make sure saved sequence\ncontains recipes that exist"
                n184 = call "Sequence Read_Write.vi"("Select"=enum16{"Save Sequence", "Read Sequence"}."Read Sequence") -> ("Sequence OUT"=w583:string[])  [unwired: 9 in, 1 out]
                n185 = for {
                  tunnel: w583 -> [w590] mode=indexing
                  tunnel: w586 -> [w589]
                  shift-right: [w587] -> w584
                  shift-left: string[] [] -> [w588]
                  n186 = for {
                    tunnel: w590 -> [w592]
                    tunnel: w589 -> [w595] mode=indexing
                    tunnel: w588 -> [w593]
                    tunnel: [w591] -> w587
                    stop <- w594 stop-if-true
                    n187 = Equal?(x=w592, y=w595) -> (x = y?=w594:bool)
                    n188 = case shown="True" w594 {
                      tunnel: w593 -> [w596 w599]
                      tunnel: w592 -> [_ w598]
                      tunnel: [w596 w597] -> w591
                      frame False {
                      }
                      frame True {
                        n189 = Build Array (concatenate)(w599, w598) -> (w597:string[])
                      }
                    }
                  }
                }
                n190 = local write "Test Trials to Run"(w584) -> ()
              }
            }
          }
          event "Reset Sequence to Default": Value Change {
            n191 = event-data() -> ()  [unwired: 1 in, 6 out]
            n192 = stacked-sequence {
              frame #0 {
                n193 = control-ref of="Test Trials to Run"() -> (w602:refnum<vi>)
                n194 = invoke class="Arr (strict)" method="Reinit To Default"(reference=w602) -> ()  [unwired: 2 in, 3 out]
              }
              frame #1 {
                w604 = refnum<vi> refnum  # ComboBox
                n195 = property on="Test Trials to Run" class="Arr (strict)"() -> ("Array Element"=w605:refnum<vi>)  [unwired: 2 in, 2 out]
                n196 = call "Trial Config - Load Filenames.vi"() -> ("Trial Config File Names OUT"=w603:string[])  [unwired: 10 in, 1 out]
                n197 = To More Specific Class(target class=w604, reference=w605) -> (specific class reference=w606:refnum<vi>)  [unwired: 1 in, 1 out]
                n198 = property class="CmbBox"(reference=w606, "Strings[]"=w603) -> ()  [unwired: 1 in, 2 out]
              }
              frame #2 {
                n199 = local write "Test Trials to Run"(string[] [] ("Test Trials to Run")) -> ()
              }
              frame #3 {
                n200 = Wait (ms)(milliseconds to wait=u32 500) -> ()  [unwired: 1 out]
              }
              frame #4 {
                n201 = local write "Reset Sequence to Default"(FALSE ("Reset Sequence to Default")) -> ()
              }
            }
          }
          event "Randomize Trials?": Value Change {
            n202 = event-data() -> ()  [unwired: 1 in, 6 out]
            n203 = case shown="True" "Randomize Trials?" {
              tunnel: [1.0 ("Numeric") 1.0 ("Numeric")] -> w611
              tunnel: [T4."Disabled and Grayed Out" ("Disabled") T4."Enabled" ("Disabled")] -> w610
              frame False {
              }
              frame True {
              }
            }
            n204 = property on="Group Size for Randomization" class="DigNum (strict)"("Value"=w611, "DisabledEnum"=w610) -> ()  [unwired: 2 in, 2 out]
          }
          event "Water Delivery": Value Change {
            n205 = event-data() -> ()  [unwired: 1 in, 6 out]
            n206 = Enqueue Element(queue=w622, element=Command."Water Delivery", error in (no error)=w621) -> (queue out=w620:refnum<queue>, error out=w619:errorcluster)  [unwired: 1 in, 1 out]
          }
          event User Event {
            n207 = event-data() -> ()  [unwired: 1 in, 4 out]
          }
          event "Log Event": Value Change {
            n208 = event-data() -> ()  [unwired: 1 in, 6 out]
            n209 = shared-variable "RT CompactRIO Target\\Shared Variables.lvlib\\Event Message to PC"() -> (w628:string)  [unwired: 1 in, 1 out]
            n210 = local write "Log Event"(FALSE ("Log Event")) -> ()
            n211 = call "Log Message.vi"("Message"=w628, "Log Type"="Event from RealTime VI") -> ()  [unwired: 8 in, 2 out]
          }
          event "Exit": Value Change {
            n212 = event-data() -> ()  [unwired: 1 in, 6 out]
            n213 = property on="Exit" class="Bool (strict)"("DisabledEnum"=T4."Disabled and Grayed Out" ("Disabled")) -> ()  [unwired: 2 in, 2 out]
            n214 = Enqueue Element(queue=w635, element=Command."Exit", error in (no error)=w634) -> (queue out=w633:refnum<queue>, error out=w632:errorcluster)  [unwired: 1 in, 1 out]
          }
        }
      }
      n215 = timed-loop {
        tunnel: w64 -> [_]
        timing: w61 -> [_]
        timing-out: [_] -> w60
        stop <- "Exit" stop-if-true
        # "Update Loop"
        n216 = node-c288() -> (w110:i64)  [unwired: 1 in, 1 out]
        n217 = local read "Start Test"() -> (w105:bool)
        n218 = call "Ball Speed Graph Accumulator.vi"("Start Test"=w105) -> ("cor_pos"=→"cor_pos":sgl, "Vball"=→"Vball":dbl, "lat_ball_motion"=→"lat_ball_motion":dbl, "for_ball_motion"=→"for_ball_motion":dbl, "Total Test Time"=w111:dbl, "Chart Ball Speed"=w112:cluster{dbl[], dbl[]}[])  [unwired: 5 in]
        "Total Test Time" <- w111
        n219 = stacked-sequence {
          tunnel: w105 -> [_ _ w129 _ w137 _ _ _ _ _ _ _]
          frame #0 {
            n220 = shared-variable "RT CompactRIO Target\\Shared Variables.lvlib\\Trial Fraction"() -> (→"Trial Fraction":dbl)  [unwired: 1 in, 1 out]
            n221 = shared-variable "RT CompactRIO Target\\Shared Variables.lvlib\\Trial#"() -> (→"Trial #":i16)  [unwired: 1 in, 1 out]
          }
          frame #1 {
            n222 = shared-variable "RT CompactRIO Target\\Shared Variables.lvlib\\ManualOverride"("Manual Override") -> ()  [unwired: 1 in, 1 out]
          }
          frame #2 {
            n223 = shared-variable "RT CompactRIO Target\\Shared Variables.lvlib\\Mean Velocities"() -> (w132:dbl[])  [unwired: 1 in, 1 out]
            n224 = case shown="True" w129 {
              frame False {
                n225 = shared-variable "RT CompactRIO Target\\Shared Variables.lvlib\\Analog Ouputs"("Analog Outputs") -> ()  [unwired: 1 in, 1 out]
              }
              frame True {
              }
            }
            n226 = Index Array(array=w132) -> (element #1=→"mean_for_vel":dbl, element #2=→"mean_lat_vel":dbl)  [unwired: 2 in]
          }
          frame #3 {
            n227 = shared-variable "RT CompactRIO Target\\Shared Variables.lvlib\\Frame Clock Freq"() -> (w135:dbl)  [unwired: 1 in, 1 out]
            n228 = shared-variable "RT CompactRIO Target\\Shared Variables.lvlib\\Ephys Clock Freq"() -> (w134:dbl)  [unwired: 1 in, 1 out]
            n229 = shared-variable "RT CompactRIO Target\\Shared Variables.lvlib\\Trial Tracker"() -> (→"Trial Tracker":string[][])  [unwired: 1 in, 1 out]
            n230 = local write "Ephys Clock Freq"(w134) -> ()
            n231 = local write "Frame Clock Freq"(w135) -> ()
          }
          frame #4 {
            n232 = shared-variable "RT CompactRIO Target\\Shared Variables.lvlib\\cRIO System DateTime"() -> (w138:string[])  [unwired: 1 in, 1 out]
            n233 = case shown="True" w137 {
              frame False {
              }
              frame True {
                n234 = shared-variable "RT CompactRIO Target\\Shared Variables.lvlib\\Laser Signal Timing"() -> (w143:i16[])  [unwired: 1 in, 1 out]
                n235 = Index Array(array=w143) -> (element #1=w142:i16, element #2=w141:i16)  [unwired: 2 in]
                n236 = local write "laser_OFF Time"(w141) -> ()
                n237 = local write "laser_ON Time"(w142) -> ()
              }
            }
            n238 = Index Array(array=w138) -> (element #1=→"cRIO System Date":string, element #2=→"cRIO System Time":string)  [unwired: 2 in]
          }
          frame #5 {
            n239 = shared-variable "RT CompactRIO Target\\Shared Variables.lvlib\\Ball Tracker Voltages"() -> (w147:sgl[])  [unwired: 1 in, 1 out]
            "Analog Inputs" <- w147
            n240 = Build Array(w147) -> (w145:T3)
            n241 = Transpose Matrix(1:w145) -> (0:→"cam_vel_ai_vlt":T3)
            n242 = shared-variable "RT CompactRIO Target\\Shared Variables.lvlib\\Test Folder Name"() -> (→"Test Folder":string)  [unwired: 1 in, 1 out]
          }
          frame #6 {
            n243 = shared-variable "RT CompactRIO Target\\Shared Variables.lvlib\\New Event Log Entry"() -> (w150:bool)  [unwired: 1 in, 1 out]
            n244 = while {
              shift-right: [w154] -> _
              shift-left: _ -> [w156]
              tunnel: w150 -> [w154]
              tunnel: [w155] -> w149
              tunnel: [w154] -> w148
              stop <- TRUE stop-if-true
              n245 = Not Equal?(x=w156, y=w154) -> (x != y?=w155:bool)
            }
            n246 = case shown="True" w149 {
              tunnel: w148 -> [_ w151]
              frame False {
              }
              frame True {
                n247 = case shown="True" w151 {
                  frame False {
                  }
                  frame True {
                    n248 = shared-variable "RT CompactRIO Target\\Shared Variables.lvlib\\New Event Log Entry"(FALSE ("New Event Log Entry")) -> ()  [unwired: 1 in, 1 out]
                    n249 = property on="Log Event" class="Bool (strict)"("Val(Sgnl)"=TRUE ("Value (Signaling)")) -> ()  [unwired: 2 in, 2 out]
                  }
                }
              }
            }
          }
          frame #7 {
            n250 = shared-variable "RT CompactRIO Target\\Shared Variables.lvlib\\cam_vel_steps"() -> (w160:dbl[])  [unwired: 1 in, 1 out]
            n251 = Build Array(w160) -> (w158:T3)
            n252 = Transpose Matrix(1:w158) -> (0:→"cam_vel_steps":T3)
          }
          frame #8 {
            n253 = shared-variable "RT CompactRIO Target\\Shared Variables.lvlib\\Test Trial In Progress"() -> (→"Test Trial In Progress":string)  [unwired: 1 in, 1 out]
            n254 = shared-variable "RT CompactRIO Target\\Shared Variables.lvlib\\Watchdog Status"() -> (→"Watchdog Status":string)  [unwired: 1 in, 1 out]
          }
          frame #9 {
            n255 = shared-variable "RT CompactRIO Target\\Shared Variables.lvlib\\Real Time Running?"() -> (→"Real-Time Running?":bool)  [unwired: 1 in, 1 out]
            n256 = shared-variable "RT CompactRIO Target\\Shared Variables.lvlib\\Timeout Timer"() -> (→"Timeout Timer":dbl)  [unwired: 1 in, 1 out]
          }
          frame #10 {
            n257 = shared-variable "RT CompactRIO Target\\Shared Variables.lvlib\\Time Into Trial"() -> (→"Time Into Trial":dbl)  [unwired: 1 in, 1 out]
            n258 = shared-variable "RT CompactRIO Target\\Shared Variables.lvlib\\DIO"() -> (→"DIO":bool[])  [unwired: 1 in, 1 out]
          }
          frame #11 {
            n259 = shared-variable "RT CompactRIO Target\\Shared Variables.lvlib\\# water"() -> (w173:i32)  [unwired: 1 in, 1 out]
            n260 = shared-variable "RT CompactRIO Target\\Shared Variables.lvlib\\Analog Inputs_Override"("Analog Inputs_Override") -> ()  [unwired: 1 in, 1 out]
            n261 = shared-variable "RT CompactRIO Target\\Shared Variables.lvlib\\cor_width"() -> (→"cor_width" →"cor_width 2":sgl)  [unwired: 1 in, 1 out]
            n262 = local write "# water"(w173) -> ()
            n263 = shared-variable "RT CompactRIO Target\\Shared Variables.lvlib\\Wall_Positions"() -> (w171:dbl[])  [unwired: 1 in, 1 out]
            n264 = Index Array(array=w171) -> (element #1=w170:dbl, element #2=w169:dbl)  [unwired: 2 in]
            "LeftWall" <- w170
            "RightWall" <- w169
            n265 = Add(x=w170, y=w169) -> (x+y=→"Cor_width_actual":dbl)
          }
        }
        n266 = call "Trial Distance Graph Accumulator.vi"("Start Test"=w105, "Seconds of history:"="History (Seconds):", "Period(ms)"=w110) -> ("LatestPoint"=w108:cluster{"X":dbl, "Y":dbl}, "Graph OUT"=w106:cluster{"X":dbl, "Y":dbl}[])  [unwired: 6 in, 1 out]
        n267 = call "Elapsed Time"("Time Target (s)"="Graph Update Interval") -> ("Time has Elapsed"=w107:bool)  [unwired: 11 in, 7 out]
        n268 = And(x=w105, y=w107) -> (x .and. y?=w118:bool)
        n269 = case shown="True" w118 {
          tunnel: w111 -> [_ w183]
          tunnel: w105 -> [w175 _]
          tunnel: w112 -> [w176 w182]
          frame False {
            # "Falling edge"
            n270 = call "OSR_OSF.vi"("BOOL"=w175) -> ("OSF"=w174:bool)  [unwired: 9 in, 1 out]
            n271 = case shown="True" w174 {
              tunnel: w176 -> [_ w177]
              frame False {
              }
              frame True {
                n272 = local write "Chart Ball Speed"(w177) -> ()
              }
            }
          }
          frame True {
            # "Update Graphs"
            n273 = Greater?(x=w183, y="X Axis (Seconds):") -> (0:w184:bool)
            n274 = case shown="True" w184 {
              tunnel: w183 -> [_ w188]
              tunnel: "X Axis (Seconds):" -> [_ w187]
              frame False {
                n275 = property on="Chart Ball Speed" class="XYGraph (strict)"("XScale.ScaleFit"=u8 1 ("X Scale.Scale Fit")) -> ()  [unwired: 2 in, 2 out]
              }
              frame True {
                n276 = Subtract(x=w188, y=w187) -> (x-y=w186:dbl)
                n277 = property on="Chart Ball Speed" class="XYGraph (strict)"("XScale.Maximum"=w188, "XScale.Minimum"=w186, "XScale.ScaleFit"=u8 0 ("X Scale.Scale Fit")) -> ()  [unwired: 2 in, 2 out]
              }
            }
            n278 = shared-variable "RT CompactRIO Target\\Shared Variables.lvlib\\Digital Controls"() -> (w179:bool[])  [unwired: 1 in, 1 out]
            n279 = shared-variable "RT CompactRIO Target\\Shared Variables.lvlib\\Water ON Time"() -> (w180:i32)  [unwired: 1 in, 1 out]
            n280 = shared-variable "RT CompactRIO Target\\Shared Variables.lvlib\\Analog Ouputs"() -> (w181:sgl[])  [unwired: 1 in, 1 out]
            n281 = local write "Analog Outputs"(w181) -> ()
            n282 = local write "Digital Controls"(w179) -> ()
            n283 = local write "Water ON Time"(w180) -> ()
            "Chart Ball Speed" <- w182
          }
        }
        n284 = case shown="True" w107 {
          tunnel: w108 -> [_ w121]
          tunnel: w106 -> [_ w120]
          frame False {
          }
          frame True {
            n285 = property on="Graph X and Y Pos" class="XYGraph (strict)"("Active Plot"=u32 0, "Cursor.Cursor Position"=w121) -> ()  [unwired: 2 in, 2 out]
            "Graph X and Y Pos" <- w120
          }
        }
        n286 = node-c288() -> ()  [unwired: 1 in, 1 out]
      }
      n287 = while {
        shift-right: [w195] -> _
        shift-left: w68 -> [w201]
        shift-right: [w194] -> w65
        shift-left: w64 -> [w200]
        stop <- w198 stop-if-true
        # "Consumer Loop"
        n288 = Dequeue Element(queue=w201, error in (no error)=w200) -> (queue out=w197:refnum<queue>, element=w199:T1, error out=w196:errorcluster)  [unwired: 1 in, 1 out]
        n289 = case shown="No Error" w196 {
          tunnel: w199 -> [w207 _]
          tunnel: [w206 TRUE] -> w198
          tunnel: w197 -> [w205 w420]
          tunnel: w196 -> [w203 w419]
          tunnel: [w204 w418] -> w195
          tunnel: [w202 w417] -> w194
          frame No Error {
            n290 = case shown="\"Download All Trials to RT\"" w207 {
              tunnel: [_ _ _ _ _ _ _ TRUE] -> w206
              tunnel: w205 -> [w229 w303 w318 w365 w377 w387 w404 w413]
              tunnel: [w223 w301 w318 w365 w377 w387 w404 w413] -> w204
              tunnel: w203 -> [w228 w302 w317 w364 w376 w386 w403 w412]
              tunnel: [w222 w300 w317 w364 w376 w386 w403 w412] -> w202
              frame "Initialize", Default {
                n291 = local read "Randomize Trials?"() -> (w208:bool)
                n292 = case shown="True" w208 {
                  tunnel: [1.0 ("Numeric") 1.0 ("Numeric")] -> w210
                  tunnel: [T4."Disabled and Grayed Out" ("Disabled") T4."Enabled" ("Disabled")] -> w209
                  frame False {
                  }
                  frame True {
                  }
                }
                n293 = call <vilib>:"System Exec.vi"("run minimized? (F)"=TRUE, "wait until completion? (T)"=FALSE, "command line"="net use U: http://NI-cRIO-9045-01D7CF99/files /u:admin") -> ("error out"=w219:errorcluster, "standard output"=→"Drive Reconnect Message":string)  [unwired: 5 in, 2 out]
                n294 = property on="Timeout Timer" class="DigNum (strict)"("Blinking"=FALSE) -> ()  [unwired: 2 in, 2 out]
                n295 = property on="Send Digital Signals to FPGA" class="Bool (strict)"("DisabledEnum"=T4."Disabled and Grayed Out" ("Disabled")) -> ()  [unwired: 2 in, 2 out]
                n296 = call <vilib>:"Clear Errors.vi"("error in (no error)"=w219) -> ()  [unwired: 5 in, 2 out]
                n297 = local write "Test Folder"("") -> ()
                n298 = local read "Slide"() -> (w213:dbl)
                n299 = property on="XY Graph" class="XYGraph (strict)"("Active Cursor"=u32 0, "Cursor.Cursor X"=w213, "Cursor.Cursor Y"=-10.0 ("Cursor.Cursor Position:Cursor Y")) -> ()  [unwired: 2 in, 2 out]
                n300 = property on="Group Size for Randomization" class="DigNum (strict)"("Value"=w210, "DisabledEnum"=w209) -> ()  [unwired: 2 in, 2 out]
                n301 = Enqueue Element(queue=w229, element=Command."Rig Config Read", error in (no error)=w228) -> (queue out=w224:refnum<queue>, error out=w225:errorcluster)  [unwired: 1 in, 1 out]
                n302 = stacked-sequence {
                  seq-local: [w260 _] -> [_ w272]
                  frame #0 {
                    w265 = refnum<vi> refnum  # ComboBox
                    n303 = control-ref of="Test Trials to Run"() -> (w266:refnum<vi>)
                    n304 = invoke class="Arr (strict)" method="Reinit To Default"(reference=w266) -> (error out=w262:errorcluster)  [unwired: 2 in, 2 out]
                    n305 = property on="Test Trials to Run" class="Arr (strict)"(error in=w262) -> (error out=w261:errorcluster, "Array Element"=w264:refnum<vi>)  [unwired: 1 in, 1 out]
                    n306 = call "Trial Config - Load Filenames.vi"() -> ("Trial Config File Names OUT"=w260:string[])  [unwired: 10 in, 1 out]
                    n307 = To More Specific Class(target class=w265, reference=w264) -> (specific class reference=w263:refnum<vi>)  [unwired: 1 in, 1 out]
                    n308 = property class="CmbBox"(reference=w263, error in=w261, "Strings[]"=w260) -> ()  [unwired: 2 out]
                  }
                  frame #1 {
                    # "make sure saved sequence\ncontains Trial Configs that exist"
                    n309 = call "Sequence Read_Write.vi"("Trial or Rig"=enum16{"Trial", "Rig"}."Trial", "Select"=enum16{"Save Sequence", "Read Sequence"}."Read Sequence") -> ("Sequence OUT"=w269:string[])  [unwired: 8 in, 1 out]
                    n310 = for {
                      tunnel: w269 -> [w276] mode=indexing
                      tunnel: w272 -> [w275]
                      shift-right: [w273] -> w270
                      shift-left: string[] [] -> [w274]
                      n311 = for {
                        tunnel: w276 -> [w278]
                        tunnel: w275 -> [w281] mode=indexing
                        tunnel: w274 -> [w279]
                        tunnel: [w277] -> w273
                        stop <- w280 stop-if-true
                        n312 = Equal?(x=w278, y=w281) -> (x = y?=w280:bool)
                        n313 = case shown="True" w280 {
                          tunnel: w279 -> [w282 w285]
                          tunnel: w278 -> [_ w284]
                          tunnel: [w282 w283] -> w277
                          frame False {
                          }
                          frame True {
                            n314 = Build Array (concatenate)(w285, w284) -> (w283:string[])
                          }
                        }
                      }
                    }
                    n315 = local write "Test Trials to Run"(w270) -> ()
                  }
                }
                n316 = stacked-sequence {
                  seq-local: [w234 _] -> [_ w243]
                  frame #0 {
                    w236 = refnum<vi> refnum  # ComboBox
                    n317 = control-ref of="Test Rig Settings"() -> (w235:refnum<vi>)
                    n318 = invoke class="Arr (strict)" method="Reinit To Default"(reference=w235) -> (error out=w239:errorcluster)  [unwired: 2 in, 2 out]
                    n319 = property on="Test Rig Settings" class="Arr (strict)"(error in=w239) -> (error out=w240:errorcluster, "Array Element"=w237:refnum<vi>)  [unwired: 1 in, 1 out]
                    n320 = call "Rig Config - Load Filenames.vi"() -> ("Rig Config File Names OUT"=w234:string[])  [unwired: 10 in, 1 out]
                    n321 = To More Specific Class(target class=w236, reference=w237) -> (specific class reference=w238:refnum<vi>)  [unwired: 1 in, 1 out]
                    n322 = property class="CmbBox"(reference=w238, error in=w240, "Strings[]"=w234) -> ()  [unwired: 2 out]
                  }
                  frame #1 {
                    # "make sure saved sequence\ncontains Rig Configs that exist"
                    n323 = call "Sequence Read_Write.vi"("Trial or Rig"=enum16{"Trial", "Rig"}."Rig", "Select"=enum16{"Save Sequence", "Read Sequence"}."Read Sequence") -> ("Sequence OUT"=w245:string[])  [unwired: 8 in, 1 out]
                    n324 = for {
                      tunnel: w245 -> [w250] mode=indexing
                      tunnel: w243 -> [w249]
                      shift-right: [w247] -> w241
                      shift-left: string[] [] -> [w248]
                      n325 = for {
                        tunnel: w250 -> [w252]
                        tunnel: w249 -> [w255] mode=indexing
                        tunnel: w248 -> [w253]
                        tunnel: [w251] -> w247
                        stop <- w254 stop-if-true
                        n326 = Equal?(x=w252, y=w255) -> (x = y?=w254:bool)
                        n327 = case shown="True" w254 {
                          tunnel: w253 -> [w256 w259]
                          tunnel: w252 -> [_ w258]
                          tunnel: [w256 w257] -> w251
                          frame False {
                          }
                          frame True {
                            n328 = Build Array (concatenate)(w259, w258) -> (w257:string[])
                          }
                        }
                      }
                    }
                    n329 = local write "Test Rig Settings"(w241) -> ()
                  }
                }
                n330 = Enqueue Element(queue=w224, element=Command."Update Folder Tree", error in (no error)=w225) -> (queue out=w223:refnum<queue>, error out=w222:errorcluster)  [unwired: 1 in, 1 out]
              }
              frame "Start Test" {
                w299 = T1[] [enum."Download All Trials to RT"] items=["Initialize", "Start Test", "Download All Trials to RT", "Water Delivery", "Rig Config Read", "cRIO Test Data Directory", "Update Folder Tree", "Log Event", "Abort", "Exit"]
                n331 = local read "Test Trials to Run"() -> (w292:string[])
                n332 = shared-variable "RT CompactRIO Target\\Shared Variables.lvlib\\Group Size for Randomization"("Group Size for Randomization") -> ()  [unwired: 1 in, 1 out]
                n333 = shared-variable "RT CompactRIO Target\\Shared Variables.lvlib\\Test Trial File Name List"(w292) -> ()  [unwired: 1 in, 1 out]
                n334 = property on="Histogram Plot1" class="Ring (strict)"("Strings []"=w292, "Value"=0 ("index")) -> ()  [unwired: 2 in, 2 out]
                n335 = property on="Histogram Plot2" class="Ring (strict)"("Strings []"=w292, "Value"=1 ("index")) -> ()  [unwired: 2 in, 2 out]
                n336 = shared-variable "RT CompactRIO Target\\Shared Variables.lvlib\\# water"(0 ("# water")) -> ()  [unwired: 1 in, 1 out]
                n337 = local read "Randomize Trials?"() -> (w287:bool)
                n338 = for {
                  shift-right: [w307] -> w301
                  shift-left: w303 -> [w308]
                  shift-right: [w305] -> w300
                  shift-left: w302 -> [w306]
                  tunnel: w299 -> [w304] mode=indexing
                  n339 = Enqueue Element(queue=w308, element=w304, error in (no error)=w306) -> (queue out=w307:refnum<queue>, error out=w305:errorcluster)  [unwired: 1 in, 1 out]
                }
                n340 = Build Array("Date", "Animal #", "Run #") -> (w295:string[])
                n341 = shared-variable "RT CompactRIO Target\\Shared Variables.lvlib\\Randomize Trials?"(w287) -> ()  [unwired: 1 in, 1 out]
                n342 = shared-variable "RT CompactRIO Target\\Shared Variables.lvlib\\Test Trial Run Array"(string[] [] ("Test Trial Run Array")) -> ()  [unwired: 1 in, 1 out]
                n343 = shared-variable "RT CompactRIO Target\\Shared Variables.lvlib\\DataFileNameVariables"(w295) -> ()  [unwired: 1 in, 1 out]
                n344 = shared-variable "RT CompactRIO Target\\Shared Variables.lvlib\\Lateral Trial History"(dbl[][] [] ("Lateral Trial History")) -> ()  [unwired: 1 in, 1 out]
                n345 = shared-variable "RT CompactRIO Target\\Shared Variables.lvlib\\Test Trial Plot Color Array"(u32[] [] ("Test Trial Plot Color Array")) -> ()  [unwired: 1 in, 1 out]
              }
              frame "Download All Trials to RT" {
                w313 = 4 ("y")
                n346 = flat-sequence {
                  tunnel: [w324] -> w316
                  frame #0 {
                    n347 = local read "Test Trials to Run"() -> (w325:string[])
                    n348 = for {
                      tunnel: w325 -> [w327] mode=indexing
                      tunnel: [w326] -> w324 mode=indexing
                      n349 = call "Read Trial Config Info.vi"("Test Trial File Name"=w327) -> ("Trial Settings OUT"=w326:T13)  [unwired: 10 in]
                    }
                    n350 = shared-variable "RT CompactRIO Target\\Shared Variables.lvlib\\Trial Cluster Array"(w324) -> ()  [unwired: 1 in, 1 out]
                  }
                  frame #1 {
                    w328 = TRUE ("Start Test")
                    n351 = shared-variable "RT CompactRIO Target\\Shared Variables.lvlib\\Start Test"(w328) -> ()  [unwired: 1 in, 1 out]
                    "Start Test" <- w328
                  }
                }
                n352 = local read "Test Trials to Run"() -> (w315:string[])
                n353 = Array Size(array=w315) -> (size(s)=w311:i32)
                n354 = for {
                  tunnel: w315 -> [w321] mode=indexing
                  tunnel: w316 -> [w323] mode=indexing
                  tunnel: [w319] -> w314
                  i -> [w322]
                  n355 = Unbundle By Name(w323) -> ("Plot Color (Lateral Dist vs Trial Fraction)"=w320:u32)
                  n356 = property on="XY Graph" class="XYGraph (strict)"("Active Plot"=w322, "Plot.Plot Name"=w321, "Plot.Plot Color"=w320) -> (error out=w319:errorcluster)  [unwired: 2 in, 1 out]
                }
                n357 = Greater Or Equal?(x=w311, y=w313) -> (x >= y?=w310:bool)
                n358 = Select(t=w313, s=w310, f=w311) -> (s? t:f=w312:i32)
                n359 = property on="XY Graph" class="XYGraph (strict)"(error in=w314, "LegNumRows"=w312, "LegScrollVis"=w310, "LegScrollPos"=u32 0 ("Legend:Scroll Position")) -> ()  [unwired: 1 in, 2 out]
              }
              frame "Rig Config Read" {
                n360 = global read "Global - Configuration Options.vi" "Rig Config Directory"() -> (w334:path)
                n361 = property on="Test Rig Config File" class="CmbBox"() -> ("Text.Text"=w345:string)  [unwired: 2 in, 2 out]
                n362 = Build Path(base path=w334, name or relative path=w345) -> (appended path=w344:path)
                n363 = call "Rig - Save or Load.vi"("RigSave Path IN"=w344, "Command IN"=Command_IN_Recipe."Load") -> ("Rig Settings OUT"=w335:T12)  [unwired: 8 in, 1 out]
                n364 = Unbundle By Name(w335) -> ("A_calib_str_row1"=w346:string, "A_calib_str_row2"=w347:string, "A_calib_str_row3"=w348:string, "Zero_V_str"=w356:string, "step_V"=w359:string, "speed_time_length"=w337:string, "Randomize Trials?"=w331:bool)
                n365 = shared-variable "RT CompactRIO Target\\Shared Variables.lvlib\\Rig Config Settings"(w335) -> ()  [unwired: 1 in, 1 out]
                n366 = Build Array(w346, w347, w348, w356) -> (w349:string[])
                n367 = Decimal String To Number(string=w337) -> (number=w336:i32)  [unwired: 2 in, 1 out]
                "Speed_Time_Length" <- w336
                n368 = Fract/Exp String To Number(string=w359) -> (number=w338:dbl)  [unwired: 3 in, 1 out]
                "step_V" <- w338
                n369 = local write "Randomize Trials?"(w331) -> ()
                n370 = for {
                  tunnel: w349 -> [w370] mode=indexing
                  tunnel: [w366] -> w355 mode=indexing
                  n371 = for {
                    N: 3 -> [_]
                    tunnel: [w372] -> w369 mode=indexing
                    shift-right: [w371] -> w368
                    shift-left: w370 -> [w374]
                    n372 = Match Pattern(string=w374, regular expression=",") -> (before substring=w372:string, after substring=w371:string)  [unwired: 1 in, 2 out]
                  }
                  n373 = Build Array (concatenate)(w369, w368) -> (w366:string[])
                }
                n374 = shared-variable "RT CompactRIO Target\\Shared Variables.lvlib\\Speed_Time_Length"(w336) -> ()  [unwired: 1 in, 1 out]
                n375 = shared-variable "RT CompactRIO Target\\Shared Variables.lvlib\\step_V"(w338) -> ()  [unwired: 1 in, 1 out]
                n376 = Select(t=T4."Enabled" ("Disabled"), s=w331, f=T4."Disabled and Grayed Out" ("Disabled")) -> (s? t:f=w332:T4)
                n377 = property on="Group Size for Randomization" class="DigNum (strict)"("DisabledEnum"=w332, "Value"=1 ("Group Size for Randomization")) -> ()  [unwired: 2 in, 2 out]
                n378 = Fract/Exp String To Number(string=w355) -> (number=w350:dbl[][])  [unwired: 3 in, 1 out]
                n379 = Index Array(array=w350) -> (element #1=w351:dbl[], element #2=w352:dbl[], element #3=w353:dbl[], element #4=w357:dbl[])  [unwired: 8 in]
                n380 = Build Array(w357) -> (w358:T3)
                n381 = Build Array(w351, w352, w353) -> (w354:T3)
                n382 = Transpose Matrix(1:w354) -> (0:w360:T3)
                "A_calib_matrix" <- w360
                n383 = Transpose Matrix(1:w358) -> (0:w339:T3)
                "zero_V" <- w339
                n384 = Index Array(array=w360, index (row) #1=0 ("index (row)"), index (row) #2=1 ("index (row)")) -> (element #1=w361:dbl[], element #2=w362:dbl[])  [unwired: 2 in]
                n385 = Index Array(array=w339, index (row)=0) -> (element=w363:dbl[])  [unwired: 1 in]
                n386 = shared-variable "RT CompactRIO Target\\Shared Variables.lvlib\\A_calib_matrix_row0"(w361) -> ()  [unwired: 1 in, 1 out]
                n387 = shared-variable "RT CompactRIO Target\\Shared Variables.lvlib\\A_calib_matrix_row1"(w362) -> ()  [unwired: 1 in, 1 out]
                n388 = shared-variable "RT CompactRIO Target\\Shared Variables.lvlib\\zero_V"(w363) -> ()  [unwired: 1 in, 1 out]
              }
              frame "Water Delivery" {
                n389 = local read "Water Delivery"() -> (w375:bool)
                n390 = case shown="True" w375 {
                  frame False {
                  }
                  frame True {
                    n391 = flat-sequence {
                      frame #0 {
                        n392 = local read "Start Test"() -> (w378:bool)
                        n393 = case shown="False" w378 {
                          frame False {
                            n394 = shared-variable "RT CompactRIO Target\\Shared Variables.lvlib\\Water ON Time"("Water ON Time") -> ()  [unwired: 1 in, 1 out]
                          }
                          frame True {
                            # "Test Is Running so no\nControl of Water Time"
                          }
                        }
                      }
                      frame #1 {
                        n395 = shared-variable "RT CompactRIO Target\\Shared Variables.lvlib\\Water Manual Reward"(TRUE ("Water Manual Reward")) -> ()  [unwired: 1 in, 1 out]
                      }
                      frame #2 {
                        n396 = Wait (ms)(milliseconds to wait=u32 200) -> ()  [unwired: 1 out]
                      }
                      frame #3 {
                        n397 = shared-variable "RT CompactRIO Target\\Shared Variables.lvlib\\# water"() -> (w382:i32)  [unwired: 1 in, 1 out]
                        n398 = local write "Water Delivery"(FALSE ("Water Delivery")) -> ()
                        n399 = Increment(x=w382) -> (x+1=w383:i32)
                        n400 = shared-variable "RT CompactRIO Target\\Shared Variables.lvlib\\# water"(w383) -> ()  [unwired: 1 in, 1 out]
                      }
                    }
                  }
                }
              }
              frame "Update Folder Tree" {
                n401 = stacked-sequence {
                  frame #0 {
                    w388 = T4."Disabled and Grayed Out" ("Disabled")
                    w389 = TRUE ("Visible")
                    n402 = property on="Flash Drive Message" class="Str"("Visible"=w389, "Blinking"=w389) -> ()  [unwired: 2 in, 2 out]
                    n403 = property on="Start Test" class="Bool (strict)"("DisabledEnum"=w388) -> ()  [unwired: 2 in, 2 out]
                    n404 = property on="Trial editor" class="Bool (strict)"("DisabledEnum"=w388) -> ()  [unwired: 2 in, 2 out]
                    n405 = property on="Rig editor" class="Bool (strict)"("DisabledEnum"=w388) -> ()  [unwired: 2 in, 2 out]
                    n406 = property on="Water Delivery" class="Bool (strict)"("DisabledEnum"=w388) -> ()  [unwired: 2 in, 2 out]
                    n407 = property on="View Event Log" class="Bool (strict)"("DisabledEnum"=w388) -> ()  [unwired: 2 in, 2 out]
                    n408 = property on="Open Flash Drive Directory" class="Bool (strict)"("DisabledEnum"=w388) -> ()  [unwired: 2 in, 2 out]
                    n409 = property on="Refresh Tree" class="Bool (strict)"("DisabledEnum"=w388) -> ()  [unwired: 2 in, 2 out]
                    n410 = property on="Exit" class="Bool (strict)"("DisabledEnum"=w388) -> ()  [unwired: 2 in, 2 out]
                    n411 = property on="Save Trial Sequence" class="Bool (strict)"("DisabledEnum"=w388) -> ()  [unwired: 2 in, 2 out]
                    n412 = property on="Load Default Sequence" class="Bool (strict)"("DisabledEnum"=w388) -> ()  [unwired: 2 in, 2 out]
                    n413 = property on="Reset Sequence to Default" class="Bool (strict)"("DisabledEnum"=w388) -> ()  [unwired: 2 in, 2 out]
                    n414 = property on="Save Rig Sequence" class="Bool (strict)"("DisabledEnum"=w388) -> ()  [unwired: 2 in, 2 out]
                  }
                  frame #1 {
                    n415 = global read "Global - Configuration Options.vi" "Rig Config Settings"() -> (w394:T12)
                    n416 = Unbundle By Name(w394) -> ("cRIO Test Data Dir"=w390:path)
                    n417 = control-ref of="Tree"() -> (w395:refnum<vi>)
                    n418 = local write "Refresh Tree"(FALSE ("Refresh Tree")) -> ()
                    n419 = call "Explorer Tree Main.vi"("error in (no error)"=errorcluster {"status"=FALSE, "code"=0, "source"=""}, "Folder Path"=w390, "TreeControl in"=w395) -> ("error out"=w392:errorcluster)  [unwired: 8 in]
                    n420 = case shown="Error" w392 {
                      tunnel: w390 -> [w396 _]
                      frame No Error {
                        n421 = call "Establish Mapped Drive Conn.vi"("Data Logging Directory IN"=w396) -> ()  [unwired: 11 in]
                      }
                      frame Error {
                        n422 = local read "Save Data"() -> (w397:bool)
                        n423 = case shown="True" w397 {
                          frame False {
                          }
                          frame True {
                            n424 = call "Flash Drive Error Conn Message.vi"() -> ()  [unwired: 12 in]
                          }
                        }
                      }
                    }
                  }
                  frame #2 {
                    w398 = FALSE ("Visible")
                    n425 = property on="Flash Drive Message" class="Str"("Visible"=w398, "Blinking"=w398) -> ()  [unwired: 2 in, 2 out]
                  }
                  frame #3 {
                    w399 = T4."Enabled" ("Disabled")
                    n426 = property on="Start Test" class="Bool (strict)"("DisabledEnum"=w399) -> ()  [unwired: 2 in, 2 out]
                    n427 = property on="Trial editor" class="Bool (strict)"("DisabledEnum"=w399) -> ()  [unwired: 2 in, 2 out]
                    n428 = property on="Rig editor" class="Bool (strict)"("DisabledEnum"=w399) -> ()  [unwired: 2 in, 2 out]
                    n429 = property on="Water Delivery" class="Bool (strict)"("DisabledEnum"=w399) -> ()  [unwired: 2 in, 2 out]
                    n430 = property on="View Event Log" class="Bool (strict)"("DisabledEnum"=w399) -> ()  [unwired: 2 in, 2 out]
                    n431 = property on="Open Flash Drive Directory" class="Bool (strict)"("DisabledEnum"=w399) -> ()  [unwired: 2 in, 2 out]
                    n432 = property on="Refresh Tree" class="Bool (strict)"("DisabledEnum"=w399) -> ()  [unwired: 2 in, 2 out]
                    n433 = property on="Exit" class="Bool (strict)"("DisabledEnum"=w399) -> ()  [unwired: 2 in, 2 out]
                    n434 = property on="Save Trial Sequence" class="Bool (strict)"("DisabledEnum"=w399) -> ()  [unwired: 2 in, 2 out]
                    n435 = property on="Load Default Sequence" class="Bool (strict)"("DisabledEnum"=w399) -> ()  [unwired: 2 in, 2 out]
                    n436 = property on="Reset Sequence to Default" class="Bool (strict)"("DisabledEnum"=w399) -> ()  [unwired: 2 in, 2 out]
                    n437 = property on="Save Rig Sequence" class="Bool (strict)"("DisabledEnum"=w399) -> ()  [unwired: 2 in, 2 out]
                  }
                }
                n438 = local write "Tab Control 2"(enum32{"Misc", "Additional Graphs"}."Misc" ("Tab Control 2")) -> ()
              }
              frame "cRIO Test Data Directory" {
                n439 = global read "Global - Configuration Options.vi" "Rig Config Settings"() -> (w401:T12)
                n440 = Unbundle By Name(w401) -> ("cRIO Test Data Dir"=w400:path)
                n441 = case shown="True" "Open Flash Drive Directory" {
                  tunnel: w400 -> [_ w405]
                  frame False {
                  }
                  frame True {
                    (unwired) path "U:/u" ("input 1")
                    # "Open windows folder of flash drive"
                    n442 = local write "Open Flash Drive Directory"(FALSE ("cRIO Test Data Directory")) -> ()
                    n443 = Format Into String(format string="cmd /c explorer.exe \"%s\"", w405) -> (resulting string=w410:string)  [unwired: 2 in, 1 out]
                    n444 = call <vilib>:"System Exec.vi"("run minimized? (F)"=FALSE, "wait until completion? (T)"=FALSE, "command line"=w410) -> ()  [unwired: 5 in, 4 out]
                  }
                }
              }
              frame "Exit" {
                n445 = disable-structure shown="Disabled" {
                  frame Disabled {
                    n446 = flat-sequence {
                      frame #0 {
                        n447 = Wait (ms)(milliseconds to wait=u32 500) -> ()  [unwired: 1 out]
                      }
                      frame #1 {
                        w416 = FALSE ("stop")
                        n448 = shared-variable "RT CompactRIO Target\\Shared Variables.lvlib\\Exit"(w416) -> ()  [unwired: 1 in, 1 out]
                        n449 = local write "Exit"(w416) -> ()
                      }
                    }
                  }
                  frame Enabled {
                  }
                }
                "Status" <- "Exiting......." ("Status")
              }
            }
          }
          frame Error {
            n450 = Flush Queue(queue=w420, error in (no error)=w419) -> (queue out=w418:refnum<queue>, error out=w417:errorcluster)  [unwired: 1 out]
            n451 = local write "Status"("Error in Consumer Loop" ("Status")) -> ()
          }
        }
      }
      n452 = xnode "Close FPGA VI Reference"("FPGA VI Reference In"=w57, "error in"=w56) -> ("error out"=w58:errorcluster)
      n453 = call <vilib>:"Simple Error Handler.vi"("error in (no error)"=w58) -> ()  [unwired: 4 in, 5 out]
      n454 = while {
        stop <- w104 stop-if-true
        # "Graph Update for Lateral Dist vs Trial Fraction"
        n455 = local read "Start Test"() -> (w98:bool)
        n456 = call "XY Graph Update.vi"("Start Test"=w98, "Enable Histogram?"="Enable Histogram?") -> ("Plot Colors OUT"=→"Plot Colors OUT":u32[], "Lateral Trial History OUT"=→"Lateral Trial History":dbl[][], "Active Plots"=→"Active Plots":i32)  [unwired: 7 in]
        n457 = Wait (ms)(milliseconds to wait=u32 1500) -> ()  [unwired: 1 out]
        n458 = local read "Exit"() -> (w104:bool)
      }
      n459 = Release Queue(queue=w74, error in (no error)=w73) -> (error out=w75:errorcluster)  [unwired: 1 in, 2 out]
      n460 = node-c288(w60) -> ()  [unwired: 1 out]
      n461 = Unregister For Events(event registration refnum=w72, error in=w75) -> (error out=w76:errorcluster)
      n462 = Destroy User Event(user event=w71, error in=w76) -> (error out=w66:errorcluster)
    }
  }
  n463 = call "Event Logger.vi"("Error IN"="Error IN", "Main VI Base Path IN"=w5) -> ("Error OUT"=w3:errorcluster)  [unwired: 5 in]
  n464 = Merge Errors(w10, w9) -> (w2:errorcluster)
  n465 = flat-sequence {
    tunnel: w2 -> [w638]
    tunnel: [w638] -> w1
    frame #0 {
      n466 = call "AccessLogStatus.vi"("Operation"=enum8{"Run", "Stop", "ReadStatus"}."Stop") -> ()  [unwired: 6 in, 1 out]
    }
  }
  n467 = disable-structure shown="Disabled" {
    frame Disabled {
      # "This code was used to stop testing if a timeout occurred due to the\nmouse not moving.  It was disabled because Yurii would like the\nnext trial to start if a timeout occurs this way."
      n468 = shared-variable "RT CompactRIO Target\\Shared Variables.lvlib\\Timeout?"() -> (w640:bool)  [unwired: 1 in, 1 out]
      n469 = while {
        shift-right: [w646] -> _
        shift-left: _ -> [w648]
        tunnel: w640 -> [w646]
        tunnel: [w647] -> w642
        tunnel: [w646] -> w641
        stop <- TRUE stop-if-true
        n470 = Not Equal?(x=w648, y=w646) -> (x != y?=w647:bool)
      }
      n471 = case shown="True" w642 {
        tunnel: w641 -> [_ w643]
        frame False {
        }
        frame True {
          n472 = case shown="True" w643 {
            frame False {
            }
            frame True {
              n473 = property on="Start Test" class="Bool (strict)"("Val(Sgnl)"=FALSE ("Value (Signaling)")) -> ()  [unwired: 2 in, 2 out]
              n474 = property on="Timeout Timer" class="DigNum (strict)"("Blinking"=TRUE) -> ()  [unwired: 2 in, 2 out]
            }
          }
        }
      }
    }
    frame Enabled {
    }
  }
  n475 = Merge Errors(w3, w1) -> (→"Error Out":errorcluster)
